vi "MainEvents.vi"() -> ()   [LabVIEW 2014]
uses:
  Commandes/Type de Mouvement PilMOT.ctl
panel:
  out "error out 2":errorcluster
  in  "Nom de base du fichier de référence Ligne à Retard":string="LigneRetard"
  in  "Nom de base du fichier de référence Miroir Troué":string="MiroirTroue"
  in  "Message":string
  in  "Nom de base du fichier de référence HeNe":string="HeNe"
  out "Axe6_Messages":u16
  out "Axe5_Messages":u16
  out "Axe4_Messages":u16
  out "Axe1_Messages":u16
  out "Axe2_Messages":u16
  out "Axe3_Messages":u16
  in  "Nom de base du fichier de références atténuateurs":string="Atténuateur"
  in  "Adresse des fichiers de référence":string="C:\\Users\\loa\\Documents\\Programmes Labview\\Moteurs Compression 5fs\\Fichiers de Référence"
  in  "STOP Moteurs":bool
  out "Adresse du PilMOT":string="ni.var.psp://localhost/OPCLib/OPC1/esbimETH_2"
  in  "stop":bool
  in  "Onglets":T1(tab)
  out "HeNe\n(µm/pas)":dbl=3.1
  out "Attenuateurs\n(µm/pas)":dbl=3.1
  out "Current LR Position \n(ps, par rapport au zéro)":dbl
  out "Butée P \n(HeNe)":bool
  out "Butée N \n(HeNe)":bool
  in  "HeNe en Butée?":bool
  in  "HeNe in?":bool
  out "PosAAtt HeNe":string
  out "HeNe":i32
  in  "HeNe Switch":bool
  out "LR (µm/pas)":dbl=3.1
  out "MT (µm/pas)":dbl=3.1
  in  "LR Deplacer":bool
  in  "LR Type Mouvement":enum16{"Absolu", "Relatif"}(ring)
  in  "LR Déplacement (µm)":dbl
  in  "MT Deplacer":bool
  in  "MT Type Mouvement":enum16{"Absolu", "Relatif"}(ring)
  in  "MT Déplacement (µm)":dbl
  in  "LR Déplacer +":bool
  in  "LR Deplacer -":bool
  in  "LR Butée +":bool
  in  "LR Butée -":bool
  in  "LR STOP mvt":bool
  in  "LR Origine ici":bool
  in  "Positions?":bool
  out "Butée P":bool[](array[boolean])
  out "Butée N":bool[](array[boolean])
  out "Position à atteindre":string[](array[string])
  in  "Actif?":bool[](array[boolean])
  in  "Att.":bool[](array[boolean])
  in  "Attenuer":bool
  out "Att. 3":i32
  out "Att. 2":i32
  out "Att. 1":i32
  in  "MT Déplacer +":bool
  in  "MT Deplacer -":bool
  in  "MT Butée +":bool
  in  "MT Butée -":bool
  in  "MT STOP mvt":bool
  in  "MT Origine ici":bool
  in  "Miroir Troué PositionCodeurEnPas":i32
  in  "Ligne à retard PositionCodeurEnPas":i32
  in  "Miroir Troué PositionTheorique":i32
  in  "Ligne à retard PositionTheorique":i32
  in  "Inversion des butées HeNe":bool=TRUE
  in  "Position HeNe":bool=TRUE
  in  "Position Laser":bool
  in  "Inversion butées":bool[](array[boolean])=[TRUE, FALSE, FALSE, FALSE]
  in  "Position Atténuateur":bool[](array[boolean])
  in  "Position Miroir":bool[](array[boolean])
  in  "Increment (mm)":dbl=0.01
  in  "Inc +":bool
  in  "Inc -":bool
  in  "Atténuateur  à référencer":T2(ring)
  in  "Set Laser":bool
  in  "Position de Référence Laser":i32
  in  "Set HeNe":bool
  in  "Position de Référence HeNe":i32
  out "Axe6_PositionTheorique":i32
  out "Axe5_PositionTheorique":i32
  out "Axe4_PositionTheorique":i32
  in  "Origine ici":bool
  in  "STOP mvt":bool
  in  "Set Atténuateur":bool
  in  "Pos. Ref. Atténuateur":i32[](array[numeric])
  in  "Set Miroir":bool
  in  "Pos. Ref. Miroir":i32[](array[numeric])
  in  "Moteur à déplacer":T3(ring)
  in  "Butée -":bool
  in  "Butée +":bool
  in  "Deplacer -":bool
  in  "Déplacer +":bool
  out "Axe3_PositionTheorique":i32
  out "Axe2_PositionTheorique":i32
  out "Axe1_PositionTheorique":i32
  out "Axe6_PositionTheorique 2":i32
  out "Axe5_PositionTheorique 2":i32
  in  "Go to ref":bool
  in  "Set ref":bool
  in  "Numéro de Pos. Ref.":T4(ring)
  in  "Ref. Tab. Origine ici":bool
  in  "Ref. Tab STOP mvt":bool
  in  "Ref. Tab Butée -":bool
  in  "Ref. Tab Butée +":bool
  in  "Ref. Tab Deplacer -":bool
  in  "Ref. Tab Déplacer +":bool
  in  "Moteur à référencer":T5(ring)
  in  "Libellés pos. de référence":string[](array[string])
  out "Positions de référence":i32[](array[numeric])
  out "Axe1_PositionTheorique 2":i32
  out "Axe2_PositionTheorique 2":i32
  out "Axe3_PositionTheorique 2":i32
  out "Axe4_PositionTheorique 2":i32
  out "error out":errorcluster
  in  "error in":errorcluster
  # "Should be working now... :D"
  # "Message Axes"
  # "Attenuation"
  # "Positions à atteindre"
  # "Positions actuelles"
  # "Att1 (M1)"
  # "Att2 (M2)"
  # "Att3 (M3)"
  # "HeNe (M4)"
  # "Position à atteindre"
  # "Position actuelle"
  # "Miroir Troué (M5)"
  # "Near Field Mirror (M6)"
  # "Position butée/position de référence atténuateurs"
  # "Position Miroir\n(butée/pos.ref.)"
  # "Position Atténuateur\n(butée/pos.ref.)"
  # "Inversion des butées\n(Normal/Inversé)"
  # "Position butée/position de référence HeNe"
  # "Positions moteurs \n(théorique, en pas)"
  # "Att. 1"
  # "Att. 2"
  # "Procédure de référencement des moteurs:"
  # "Att. 3"
  # "HeNe"
  # "Miroir Troué"
  # "1. Aller en butée -\n2. Faire le zéro\n3. Déplacer jusqu'en pos. ref\n4. Set"
  # "Delay Line"
  # "Pos. ref. Miroir\n(théorique, en pas)"
  # "Pos. ref. Atténuateur\n(théorique, en pas)"
  # "Att. 1"
  # "Att. 2"
  # "Att. 3"
  # "Pos. ref. HeNe\n(théorique, en pas)"
  # "Pos. ref. Laser\n(théorique, en pas)"
  # "HeNe"
  # "Références tous moteurs"
  # "Position actuelle"
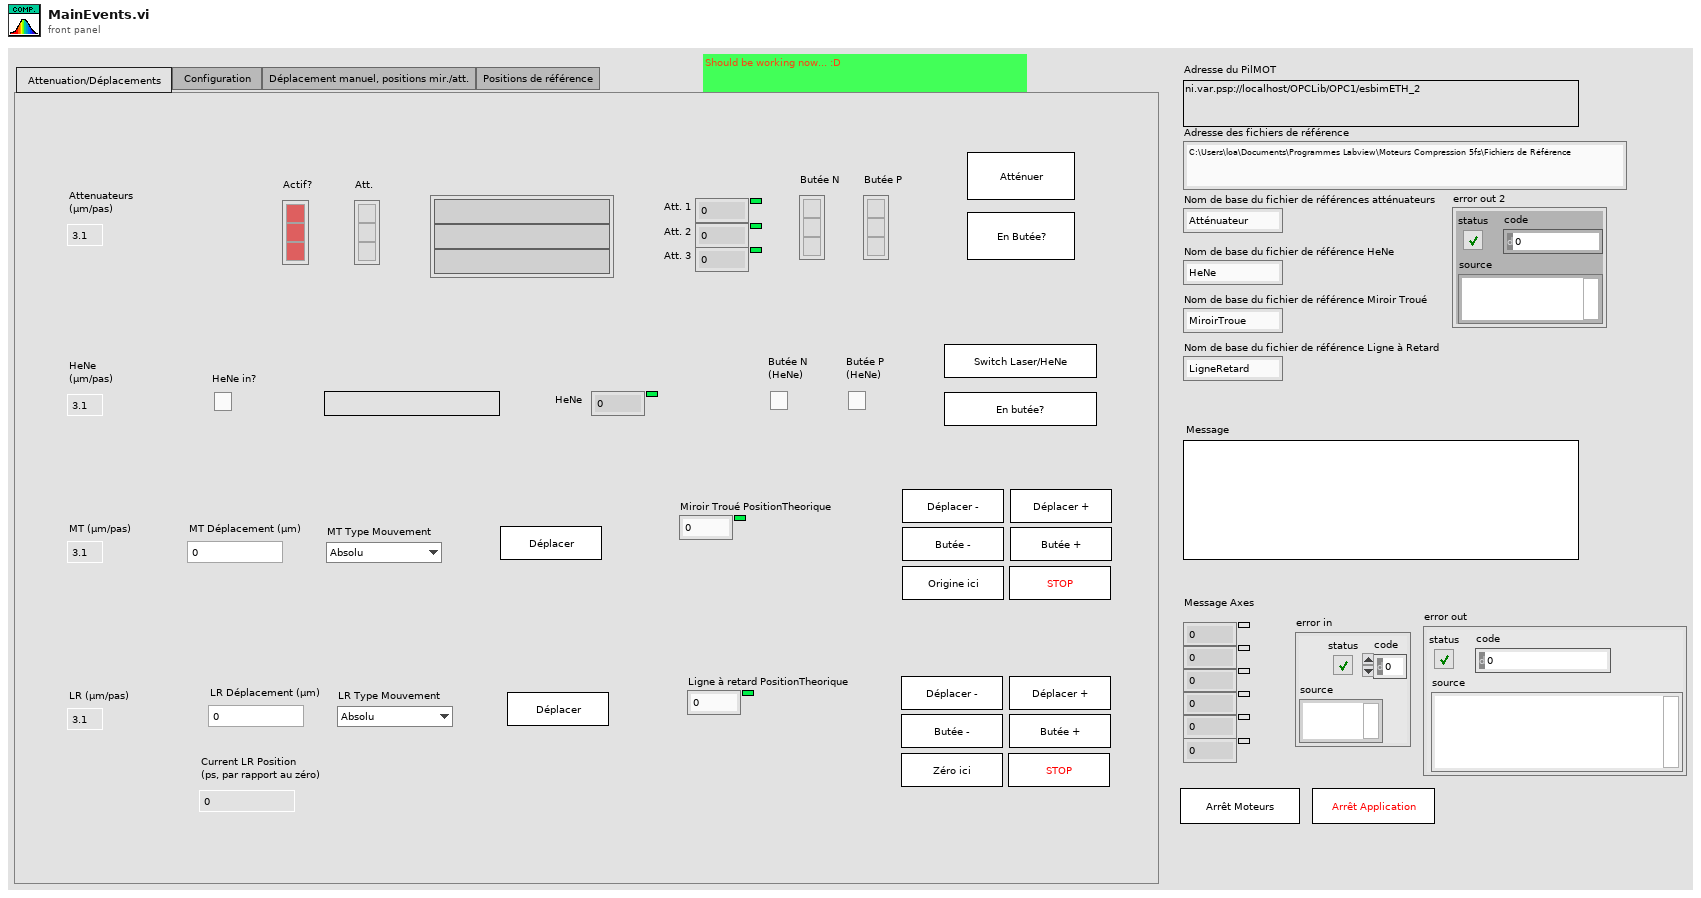
[diagram p1: front panel]
types:
  T1 = enum32{"Attenuation/Déplacements   ", "Configuration   ", "Déplacement manuel, positions mir./att.", "Positions de référence"}
  T2 = enum16{"Atténuateur 1", "Atténuateur 2", "Atténuateur 3"}
  T3 = enum16{"Atténuateur 1", "Atténuateur 2", "Atténuateur 3", "HeNe", "Miroir Troué", "Delay Line"}
  T4 = enum16{"Position 1", "Position 2", "Position 3", "Position 4"}
  T5 = enum16{"Atténuateur 1", "Atténuateur 2", "Atténuateur 3", "HeNe", "Miroir Troué", "Ligne à Retard"}
  T6 = enum16{"open", "replace", "create", "open or create", "replace or create", "replace or create with confirmation"}
  T7 = typedef "Type de Mouvement PilMOT.ctl" = u16
  T8 = typedef "AdressesVariablesPartagees.ctl" = cluster{"OrdreBloc":string, "Ordre UC":string, "CoteAAtteindre":string, "Vitesse":string, "Position codeur en pas":string, "Position Théorique":string, "Message":string, "Ecrire":string, "Zone à écrire":string, "Numéro paramètre":string, "Ordre":string, "Valeur":string, "Valeur Lecture":string, "Numéro paramètre Lecture":string, "Acquittement Lecture Ecriture":string, "Zone à Ecrire Pour Axe ":u16, "Acquittement Ordre UC":string}
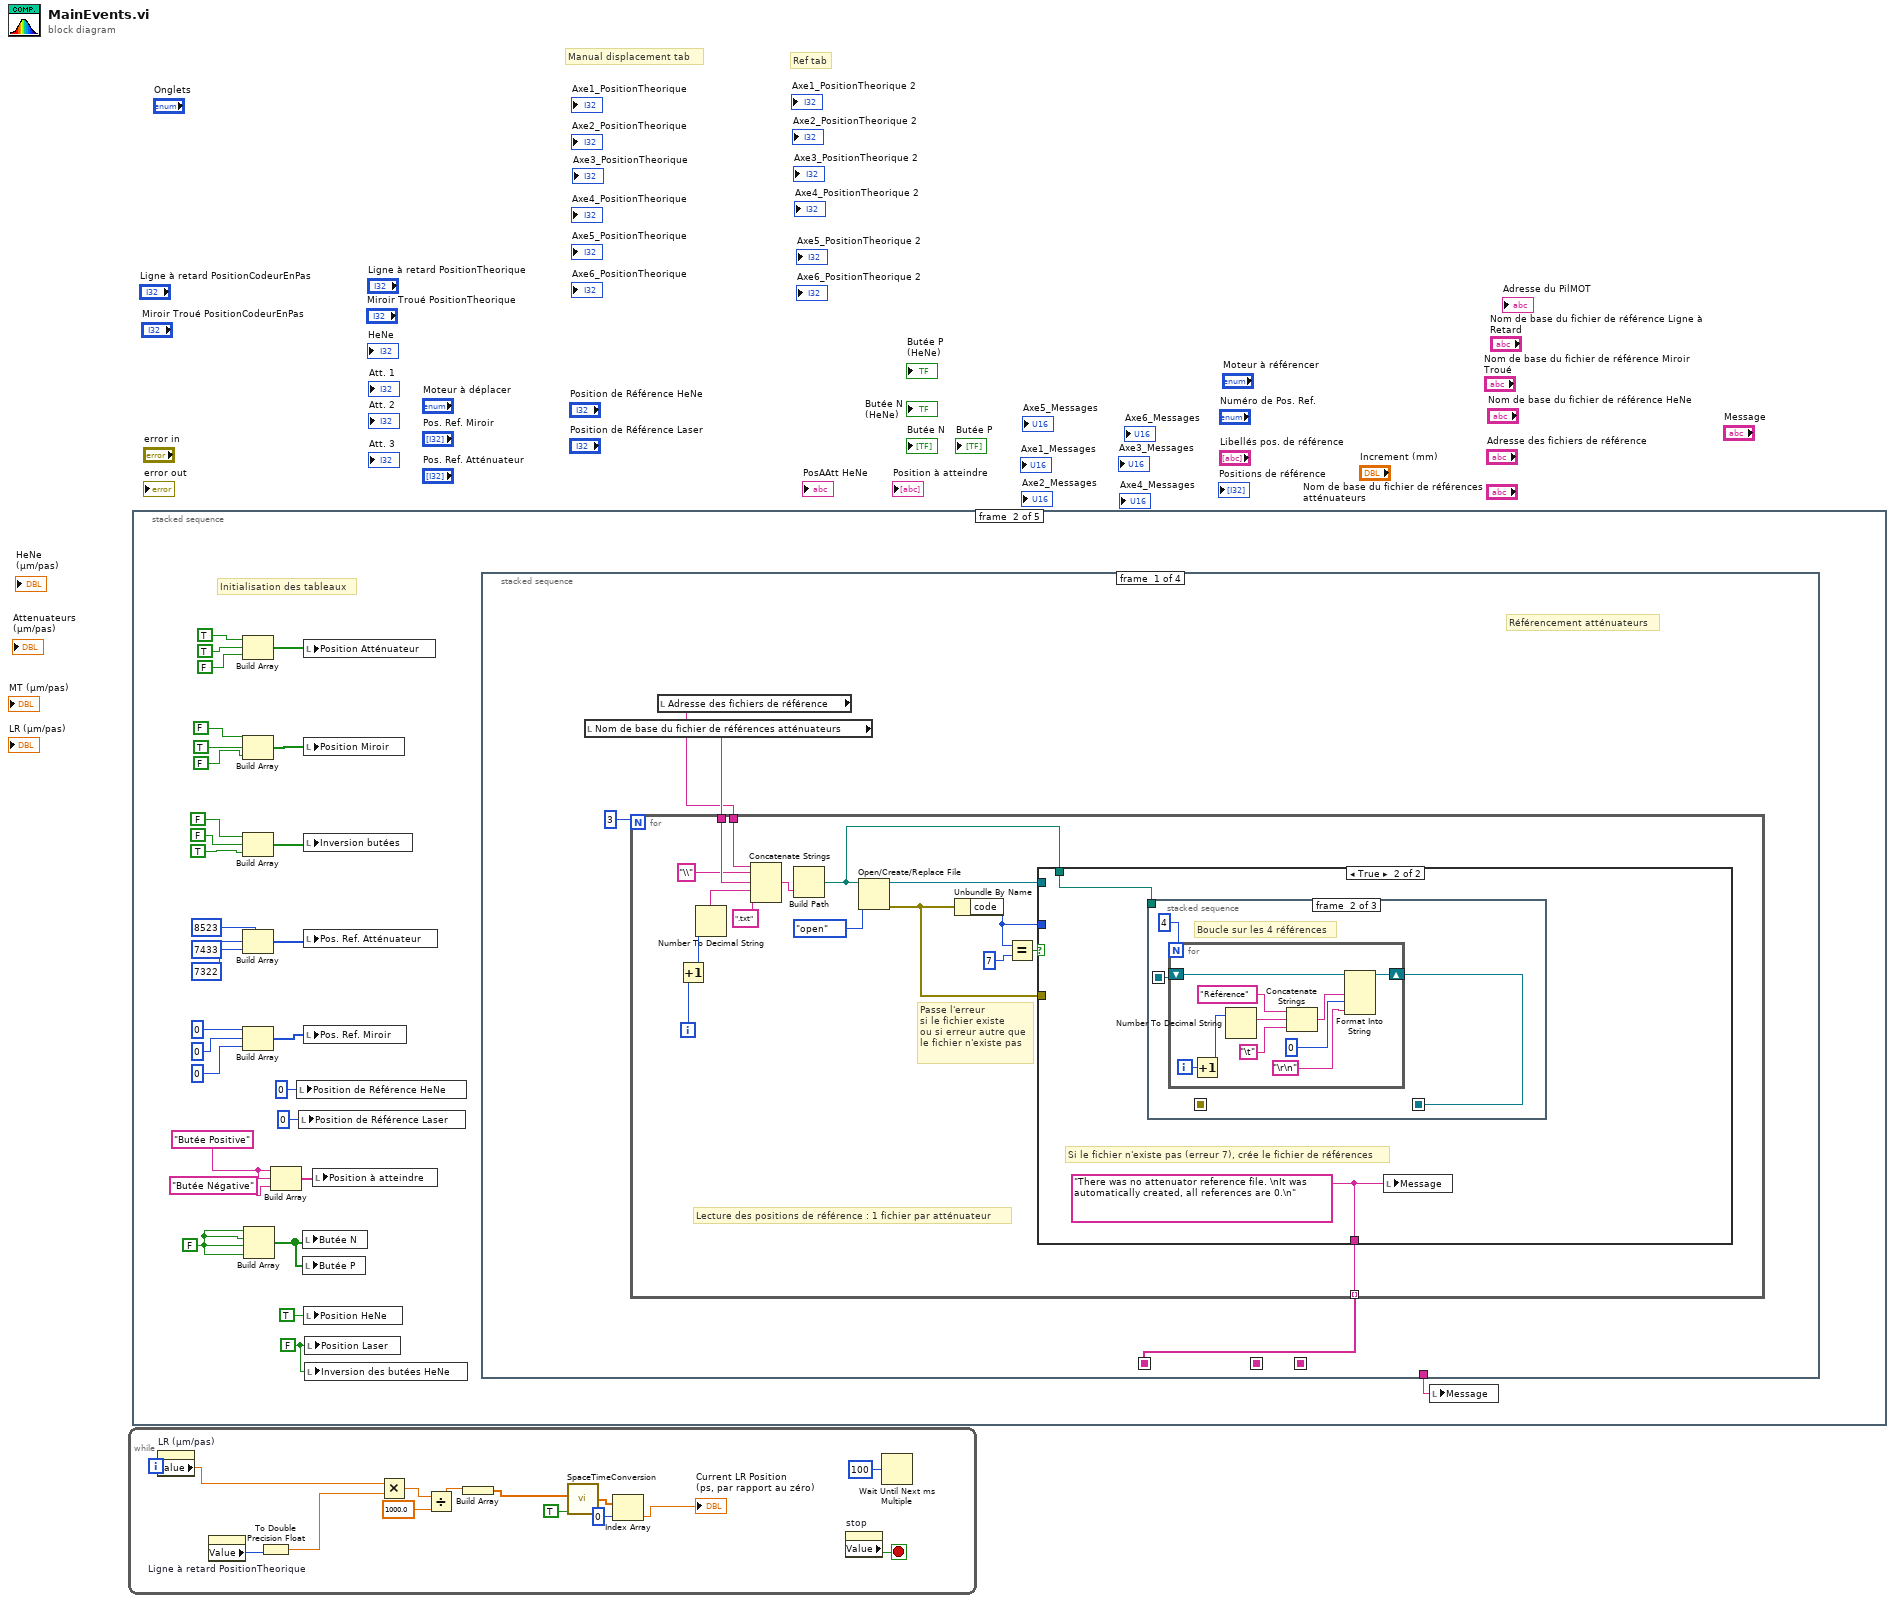
[diagram p0: block diagram]
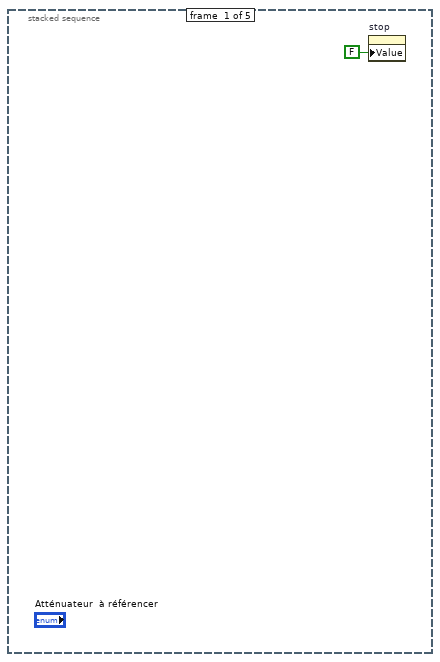
[diagram p2: hidden frame]
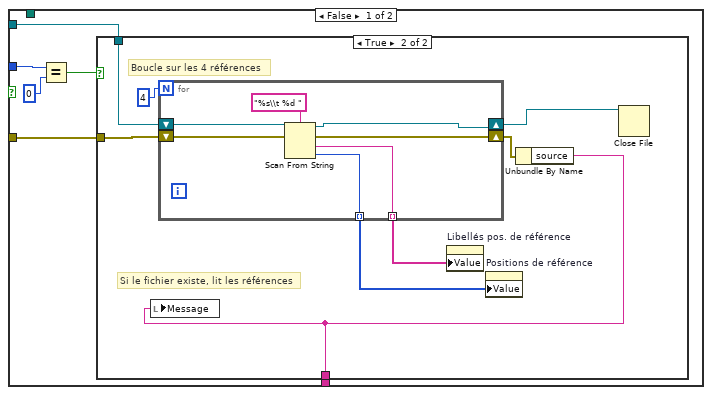
[diagram p3: hidden frame]
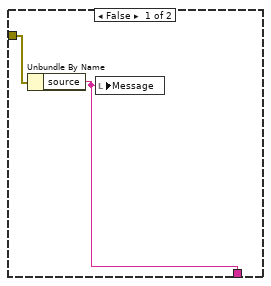
[diagram p4: hidden frame]
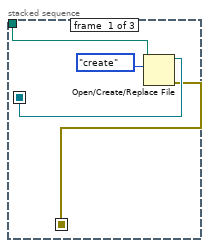
[diagram p5: hidden frame]
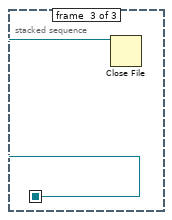
[diagram p6: hidden frame]
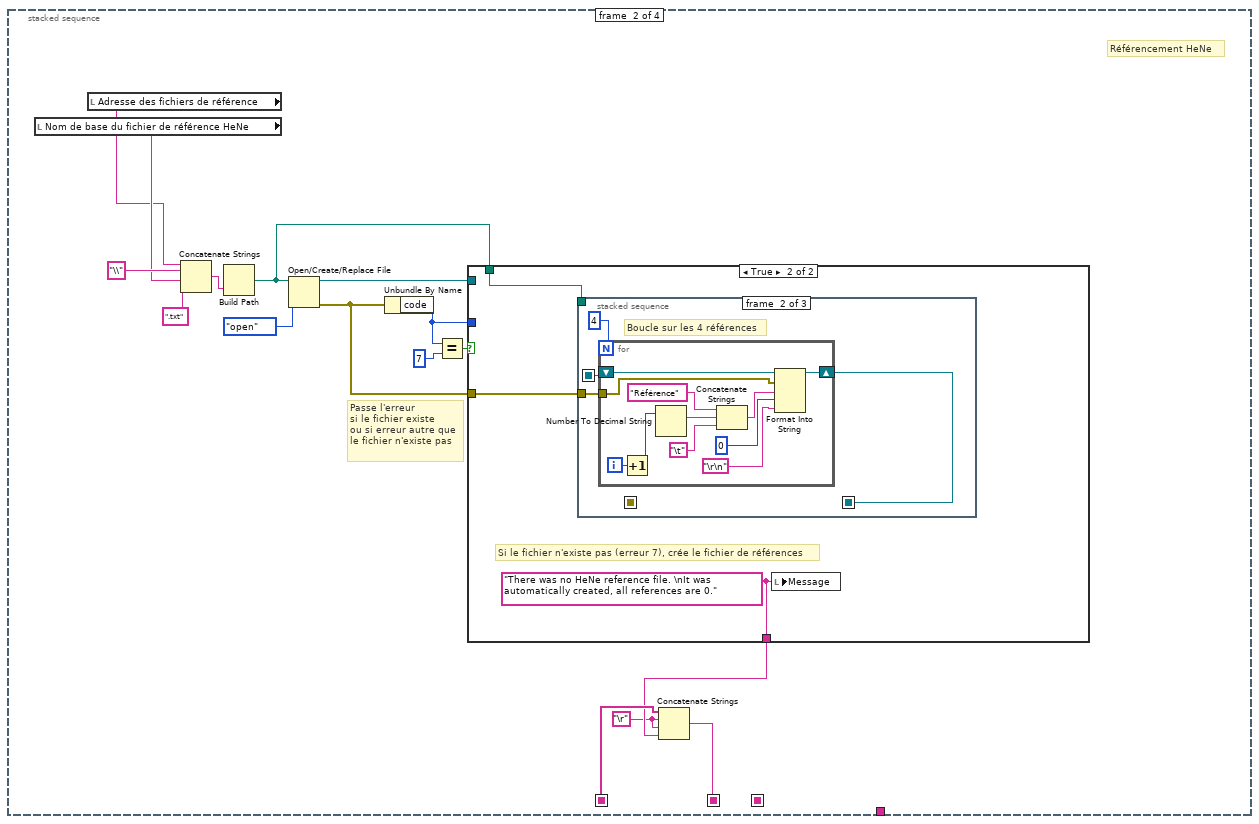
[diagram p7: hidden frame]
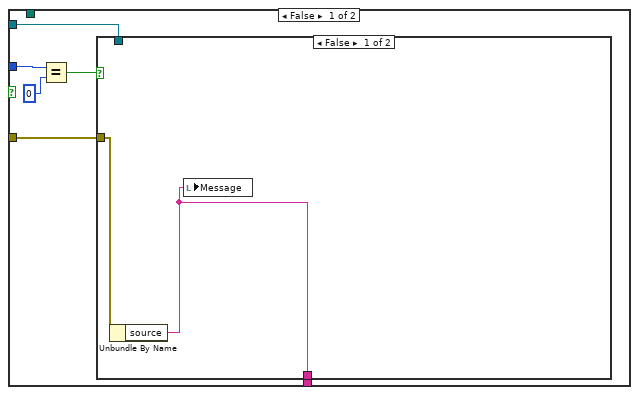
[diagram p8: hidden frame]
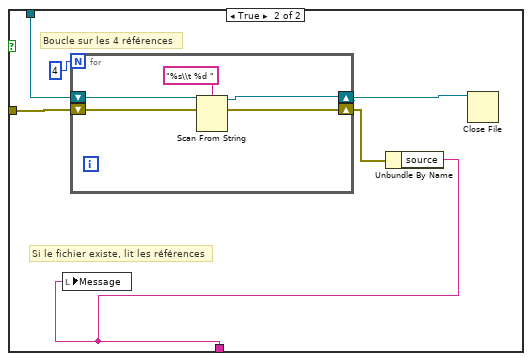
[diagram p9: hidden frame]
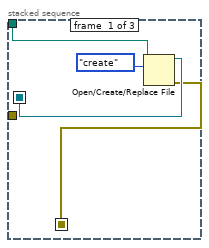
[diagram p10: hidden frame]
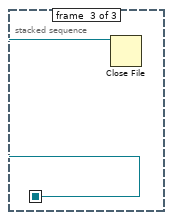
[diagram p11: hidden frame]
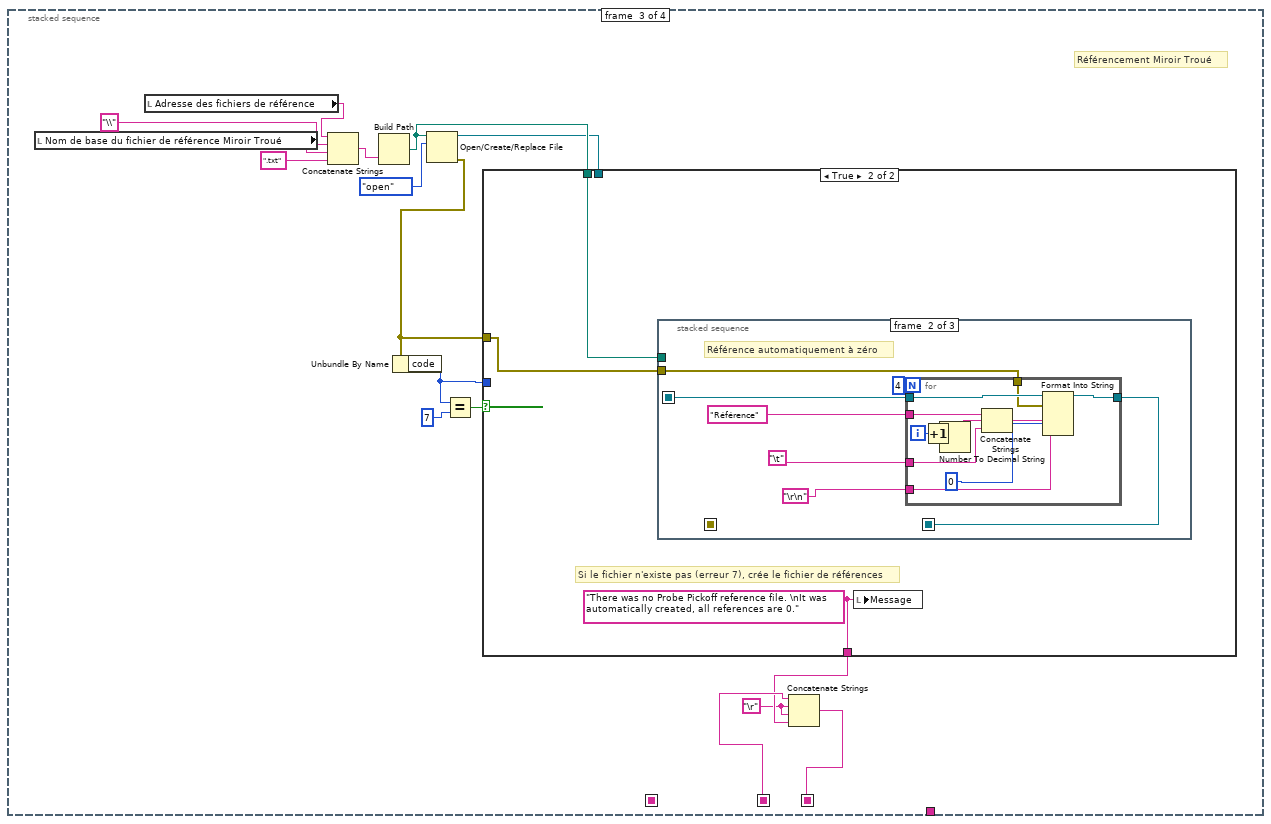
[diagram p12: hidden frame]
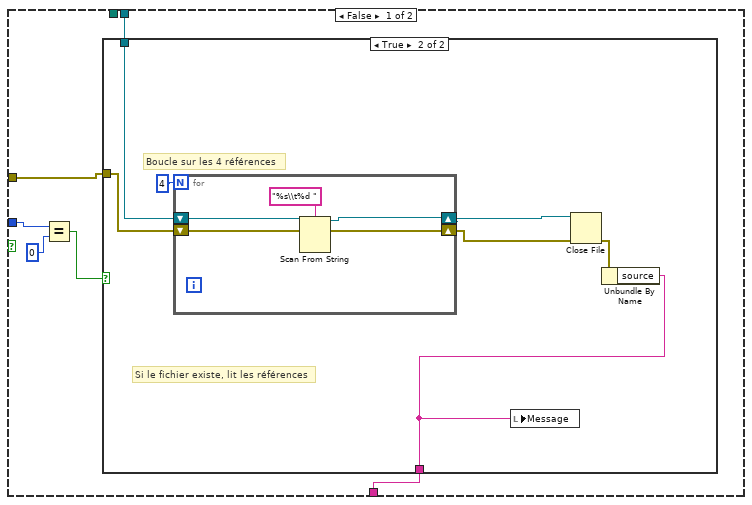
[diagram p13: hidden frame]
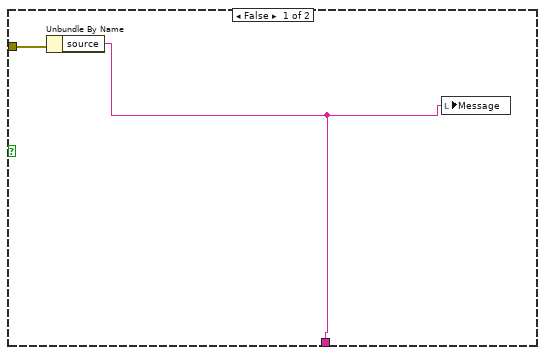
[diagram p14: hidden frame]
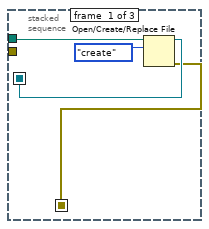
[diagram p15: hidden frame]
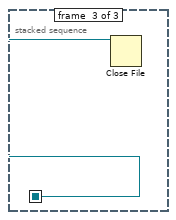
[diagram p16: hidden frame]
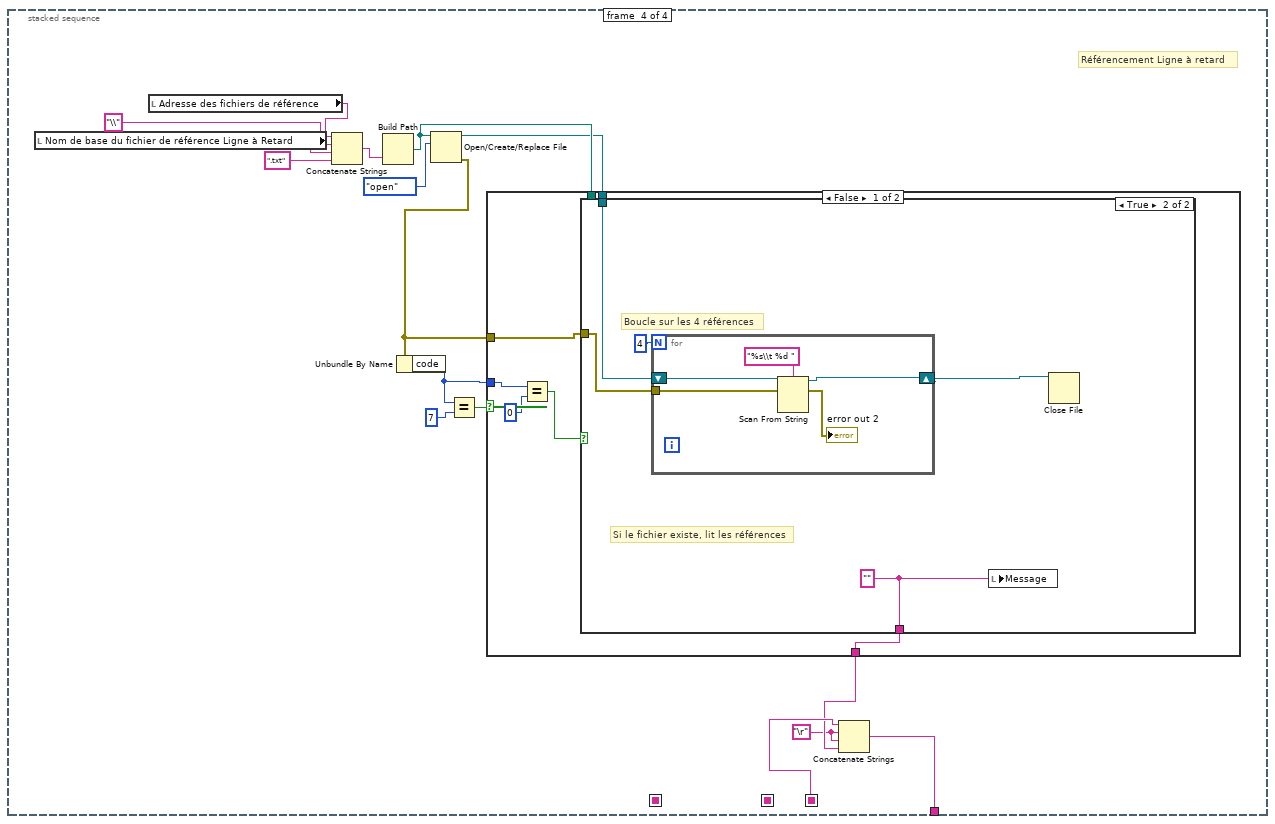
[diagram p17: hidden frame]
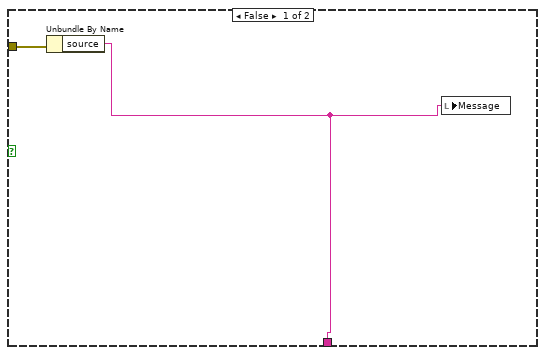
[diagram p18: hidden frame]
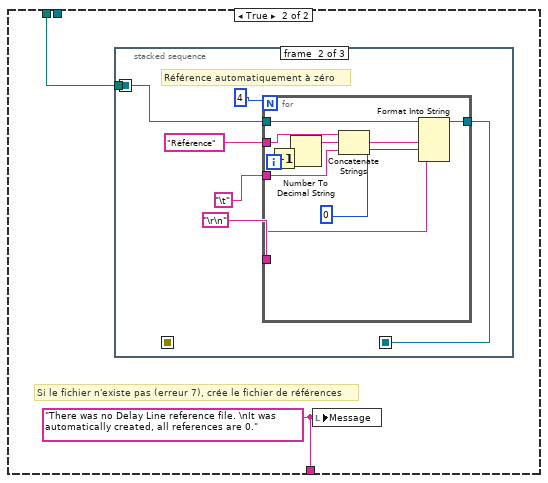
[diagram p19: hidden frame]
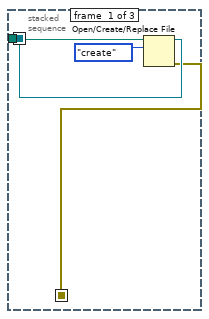
[diagram p20: hidden frame]
diagram:
  # "Ref tab"
  # "Manual displacement tab"
  n1 = while {
    stop <- w13 stop-if-true
    n2 = property on="LR (µm/pas)" class="DigNum (strict)"() -> ("Value"=w11:dbl)  [unwired: 2 in, 2 out]
    n3 = property on="Ligne à retard PositionTheorique" class="DigNum (strict)"() -> ("Value"=w10:i32)  [unwired: 2 in, 2 out]
    n4 = To Double Precision Float(number=w10) -> (double precision float=w9:dbl)
    n5 = Multiply(x=w11, y=w9) -> (x*y=w4:dbl)
    n6 = Divide(x=w4, y=1000.0) -> (x/y=w2:dbl)
    n7 = Build Array(w2) -> (w3:dbl[])
    n8 = call "SpaceTimeConversion.vi"("Conversion Type: T : Distance to Time\n                             F : Time to Distance"=TRUE ("Conversion Type: T : Distance to Time\n                             F : Time to Distance"), "Distance IN (mm)"=w3) -> ("Time OUT (ps) / Distance OUT (mm)"=w7:dbl[])  [unwired: 2 in]
    n9 = Index Array(array=w7, index=0) -> (element=→"Current LR Position \n(ps, par rapport au zéro)":dbl)
    n10 = property on="stop" class="Bool (strict)"() -> ("Value"=w13:bool)  [unwired: 2 in, 2 out]
    n11 = Wait Until Next ms Multiple(millisecond multiple=u32 100) -> ()  [unwired: 1 out]
  }
  n12 = stacked-sequence {
    frame #0 {
      n13 = property on="stop" class="Bool (strict)"("Value"=FALSE ("stop")) -> ()  [unwired: 2 in, 2 out]
    }
    frame #1 {
      w18 = FALSE ("Position Laser")
      w20 = "Butée Positive"
      w23 = FALSE
      # "Initialisation des tableaux"
      n14 = Build Array(TRUE, TRUE, FALSE) -> (w41:bool[])
      n15 = Build Array(FALSE, TRUE, FALSE) -> (w37:bool[])
      n16 = Build Array(FALSE, FALSE, TRUE) -> (w33:bool[])
      n17 = Build Array(8523, 7433, 7322) -> (w25:i32[])
      n18 = Build Array(0, 0, 0) -> (w32:i32[])
      n19 = Build Array(w23, w23, w23, w23) -> (w22:bool[])
      n20 = Build Array(w20, w20, "Butée Négative") -> (w24:string[])
      n21 = local write "Position de Référence HeNe"(0 ("Position de Référence HeNe")) -> ()
      n22 = local write "Position de Référence Laser"(0 ("Position de Référence Laser")) -> ()
      n23 = local write "Butée N"(w22) -> ()
      n24 = local write "Butée P"(w22) -> ()
      n25 = local write "Position Atténuateur"(w41) -> ()
      n26 = local write "Position Miroir"(w37) -> ()
      n27 = local write "Inversion butées"(w33) -> ()
      n28 = local write "Pos. Ref. Atténuateur"(w25) -> ()
      n29 = local write "Pos. Ref. Miroir"(w32) -> ()
      n30 = local write "Position HeNe"(TRUE ("Position HeNe")) -> ()
      n31 = local write "Position Laser"(w18) -> ()
      n32 = local write "Inversion des butées HeNe"(w18) -> ()
      n33 = local write "Position à atteindre"(w24) -> ()
      n34 = stacked-sequence {
        seq-local: [w45 _ _ _] -> [_ w111 _ _]
        seq-local: [_ w109 _ _] -> [_ _ w169 _]
        seq-local: [_ _ w167 _] -> [_ _ _ w231]
        tunnel: [_ _ _ w229] -> w15
        frame #0 {
          # "Référencement atténuateurs"
          n35 = local read "Nom de base du fichier de références atténuateurs"() -> (w47:string)
          n36 = local read "Adresse des fichiers de référence"() -> (w46:string)
          n37 = for {
            N: 3 -> [_]
            tunnel: w46 -> [w52]
            tunnel: w47 -> [w53]
            tunnel: [w49] -> w45 mode=indexing
            i -> [w64]
            # "Lecture des positions de référence : 1 fichier par atténuateur"
            # "Passe l'erreur\nsi le fichier existe\nou si erreur autre que\nle fichier n'existe pas"
            n38 = Increment(x=w64) -> (x+1=w50:i32)
            n39 = Number To Decimal String(number=w50) -> (decimal integer string=w63:string)  [unwired: 1 in]
            n40 = Concatenate Strings(w52, "\\", w53, w63, ".txt" ("string")) -> (w61:string)
            n41 = Build Path(name or relative path=w61) -> (appended path=w57:path)  [unwired: 1 in]
            n42 = Open/Create/Replace File(file path (use dialog)=w57, operation (0:open)=T6."open") -> (refnum out=w55:refnum<file>, error out=w54:errorcluster)  [unwired: 4 in, 1 out]
            n43 = Unbundle By Name(w54) -> ("code"=w56:i32)
            n44 = Equal?(x=w56, y=7) -> (x = y?=w58:bool)
            n45 = case shown="True" w58 {
              tunnel: w57 -> [_ w89]
              tunnel: w56 -> [w70 _]
              tunnel: w55 -> [w67 _]
              tunnel: w54 -> [w66 _]
              tunnel: [w65 w88] -> w49
              frame False {
                n46 = Equal?(x=w70, y=0) -> (x = y?=w68:bool)
                n47 = case shown="True" w68 {
                  tunnel: w67 -> [_ w79]
                  tunnel: w66 -> [w72 w78]
                  tunnel: [w71 w73] -> w65
                  frame False {
                    n48 = Unbundle By Name(w72) -> ("source"=w71:string)
                    n49 = local write "Message"(w71) -> ()
                  }
                  frame True {
                    # "Si le fichier existe, lit les références"
                    # "Boucle sur les 4 références"
                    n50 = for {
                      N: 4 -> [_]
                      shift-right: [w85] -> w77
                      shift-left: w79 -> [w87]
                      tunnel: [w83] -> w76 mode=indexing
                      tunnel: [w82] -> w75 mode=indexing
                      shift-right: [w81] -> w74
                      shift-left: w78 -> [w86]
                      n51 = Scan From String("%s\\t %d " ("format string"), w87, w86) -> (w85:refnum<file>, w81:errorcluster, output 1=w83:string, output 2=w82:i32)  [unwired: 2 in]
                    }
                    n52 = property on="Libellés pos. de référence" class="Arr (strict)"("Value"=w76) -> ()  [unwired: 2 in, 2 out]
                    n53 = property on="Positions de référence" class="Arr (strict)"("Value"=w75) -> ()  [unwired: 2 in, 2 out]
                    n54 = Unbundle By Name(w74) -> ("source"=w73:string)
                    n55 = local write "Message"(w73) -> ()
                    n56 = Close File(refnum=w77) -> ()  [unwired: 1 in, 2 out]
                  }
                }
              }
              frame True {
                w88 = "There was no attenuator reference file. \nIt was automatically created, all references are 0.\n" ("Message")
                # "Si le fichier n'existe pas (erreur 7), crée le fichier de références"
                n57 = stacked-sequence {
                  seq-local: [w91 _ _] -> [_ w94 _]
                  seq-local: [w90 _ _] -> [_ _ _]
                  seq-local: [_ w95 _] -> [_ _ w107]
                  tunnel: w89 -> [w93 _ _]
                  frame #0 {
                    n58 = Open/Create/Replace File(file path (use dialog)=w93, operation (0:open)=T6."create") -> (refnum out=w91:refnum<file>, error out=w90:errorcluster)  [unwired: 4 in, 1 out]
                  }
                  frame #1 {
                    # "Boucle sur les 4 références"
                    n59 = for {
                      N: 4 -> [_]
                      shift-right: [w105] -> w95
                      shift-left: w94 -> [w106]
                      i -> [w104]
                      n60 = Increment(x=w104) -> (x+1=w97:i32)
                      n61 = Number To Decimal String(number=w97) -> (decimal integer string=w103:string)  [unwired: 1 in]
                      n62 = Concatenate Strings("Référence", w103, "\t") -> (w101:string)
                      n63 = Format Into String(initial string=w106, w101, 0, "\r\n") -> (resulting string=w105:refnum<file>)  [unwired: 2 in, 1 out]
                    }
                  }
                  frame #2 {
                    n64 = Close File(refnum=w107) -> ()  [unwired: 1 in, 2 out]
                  }
                }
                n65 = local write "Message"(w88) -> ()
              }
            }
          }
        }
        frame #1 {
          w108 = "\r"
          # "Passe l'erreur\nsi le fichier existe\nou si erreur autre que\nle fichier n'existe pas"
          # "Référencement HeNe"
          n66 = local read "Nom de base du fichier de référence HeNe"() -> (w113:string)
          n67 = local read "Adresse des fichiers de référence"() -> (w112:string)
          n68 = Concatenate Strings(w112, "\\", w113, ".txt" ("string")) -> (w115:string)
          n69 = Build Path(name or relative path=w115) -> (appended path=w119:path)  [unwired: 1 in]
          n70 = Open/Create/Replace File(file path (use dialog)=w119, operation (0:open)=T6."open") -> (refnum out=w121:refnum<file>, error out=w122:errorcluster)  [unwired: 4 in, 1 out]
          n71 = Unbundle By Name(w122) -> ("code"=w120:i32)
          n72 = Equal?(x=w120, y=7) -> (x = y?=w118:bool)
          n73 = case shown="True" w118 {
            tunnel: w119 -> [_ w145]
            tunnel: w120 -> [w129 _]
            tunnel: w121 -> [w126 _]
            tunnel: w122 -> [w125 w143]
            tunnel: [w124 w144] -> w110
            frame False {
              n74 = Equal?(x=w129, y=0) -> (x = y?=w127:bool)
              n75 = case shown="False" w127 {
                tunnel: w126 -> [_ w136]
                tunnel: w125 -> [w131 w135]
                tunnel: [w130 w132] -> w124
                frame False {
                  n76 = Unbundle By Name(w131) -> ("source"=w130:string)
                  n77 = local write "Message"(w130) -> ()
                }
                frame True {
                  # "Si le fichier existe, lit les références"
                  # "Boucle sur les 4 références"
                  n78 = for {
                    N: 4 -> [_]
                    shift-right: [w140] -> w134
                    shift-left: w136 -> [w142]
                    shift-right: [w138] -> w133
                    shift-left: w135 -> [w141]
                    n79 = Scan From String("%s\\t %d " ("format string"), w142, w141) -> (w140:refnum<file>, w138:errorcluster)  [unwired: 4 in]
                  }
                  n80 = Unbundle By Name(w133) -> ("source"=w132:string)
                  n81 = local write "Message"(w132) -> ()
                  n82 = Close File(refnum=w134) -> ()  [unwired: 1 in, 2 out]
                }
              }
            }
            frame True {
              w144 = "There was no HeNe reference file. \nIt was automatically created, all references are 0." ("Message")
              # "Si le fichier n'existe pas (erreur 7), crée le fichier de références"
              n83 = stacked-sequence {
                seq-local: [w147 _ _] -> [_ w151 _]
                seq-local: [w146 _ _] -> [_ _ _]
                seq-local: [_ w152 _] -> [_ _ w165]
                tunnel: w145 -> [w149 _ _]
                tunnel: w143 -> [_ w150 _]
                frame #0 {
                  n84 = Open/Create/Replace File(file path (use dialog)=w149, operation (0:open)=T6."create") -> (refnum out=w147:refnum<file>, error out=w146:errorcluster)  [unwired: 4 in, 1 out]
                }
                frame #1 {
                  # "Boucle sur les 4 références"
                  n85 = for {
                    N: 4 -> [_]
                    shift-right: [w163] -> w152
                    shift-left: w151 -> [w164]
                    tunnel: w150 -> [w154]
                    i -> [w162]
                    n86 = Increment(x=w162) -> (x+1=w155:i32)
                    n87 = Number To Decimal String(number=w155) -> (decimal integer string=w161:string)  [unwired: 1 in]
                    n88 = Concatenate Strings("Référence", w161, "\t") -> (w159:string)
                    n89 = Format Into String(initial string=w164, error in=w154, w159, 0, "\r\n") -> (resulting string=w163:refnum<file>)  [unwired: 1 in, 1 out]
                  }
                }
                frame #2 {
                  n90 = Close File(refnum=w165) -> ()  [unwired: 1 in, 2 out]
                }
              }
              n91 = local write "Message"(w144) -> ()
            }
          }
          n92 = Concatenate Strings(w111, w108, w108, w110) -> (w109:string)
        }
        frame #2 {
          w166 = "\r"
          # "Référencement Miroir Troué"
          n93 = local read "Nom de base du fichier de référence Miroir Troué"() -> (w179:string)
          n94 = local read "Adresse des fichiers de référence"() -> (w181:string)
          n95 = Concatenate Strings(w181, "\\", w179, ".txt" ("string")) -> (w177:string)
          n96 = Build Path(name or relative path=w177) -> (appended path=w173:path)  [unwired: 1 in]
          n97 = Open/Create/Replace File(file path (use dialog)=w173, operation (0:open)=T6."open") -> (refnum out=w171:refnum<file>, error out=w170:errorcluster)  [unwired: 4 in, 1 out]
          n98 = Unbundle By Name(w170) -> ("code"=w172:i32)
          n99 = Equal?(x=w172, y=7) -> (x = y?=w174:bool)
          n100 = case shown="True" w174 {
            tunnel: w173 -> [_ w204]
            tunnel: w172 -> [w186 _]
            tunnel: w171 -> [w184 _]
            tunnel: w170 -> [w183 w202]
            tunnel: [w182 w203] -> w168
            frame False {
              n101 = Equal?(x=w186, y=0) -> (x = y?=w185:bool)
              n102 = case shown="True" w185 {
                tunnel: w184 -> [_ w195]
                tunnel: w183 -> [w189 w193]
                tunnel: [w188 w190] -> w182
                frame False {
                  n103 = Unbundle By Name(w189) -> ("source"=w188:string)
                  n104 = local write "Message"(w188) -> ()
                }
                frame True {
                  # "Si le fichier existe, lit les références"
                  # "Boucle sur les 4 références"
                  n105 = for {
                    N: 4 -> [_]
                    shift-right: [w200] -> w194
                    shift-left: w195 -> [w201]
                    shift-right: [w197] -> w192
                    shift-left: w193 -> [w198]
                    n106 = Scan From String("%s\\t%d " ("format string"), w201, w198) -> (w200:refnum<file>, w197:errorcluster)  [unwired: 4 in]
                  }
                  n107 = Close File(refnum=w194, error in=w192) -> (error out=w191:errorcluster)  [unwired: 1 out]
                  n108 = Unbundle By Name(w191) -> ("source"=w190:string)
                  n109 = local write "Message"(w190) -> ()
                }
              }
            }
            frame True {
              w203 = "There was no Probe Pickoff reference file. \nIt was automatically created, all references are 0." ("Message")
              # "Si le fichier n'existe pas (erreur 7), crée le fichier de références"
              n110 = stacked-sequence {
                seq-local: [w207 _ _] -> [_ w214 _]
                seq-local: [w206 _ _] -> [_ _ _]
                seq-local: [_ w215 _] -> [_ _ w227]
                tunnel: w204 -> [w205 _ _]
                tunnel: w202 -> [_ w209 _]
                frame #0 {
                  n111 = Open/Create/Replace File(file path (use dialog)=w205, operation (0:open)=T6."create") -> (refnum out=w207:refnum<file>, error out=w206:errorcluster)  [unwired: 4 in, 1 out]
                }
                frame #1 {
                  # "Référence automatiquement à zéro"
                  n112 = for {
                    N: 4 -> [_]
                    tunnel: [w226] -> w215
                    tunnel: w214 -> [w225]
                    tunnel: "\r\n" -> [w222]
                    tunnel: "Référence" -> [w219]
                    tunnel: "\t" -> [w217]
                    tunnel: w209 -> [w216]
                    i -> [w224]
                    n113 = Increment(x=w224) -> (x+1=w221:i32)
                    n114 = Number To Decimal String(number=w221) -> (decimal integer string=w220:string)  [unwired: 1 in]
                    n115 = Concatenate Strings(w219, w220, w217) -> (w218:string)
                    n116 = Format Into String(initial string=w225, error in=w216, w218, 0, w222) -> (resulting string=w226:refnum<file>)  [unwired: 1 in, 1 out]
                  }
                }
                frame #2 {
                  n117 = Close File(refnum=w227) -> ()  [unwired: 1 in, 2 out]
                }
              }
              n118 = local write "Message"(w203) -> ()
            }
          }
          n119 = Concatenate Strings(w169, w166, w166, w168) -> (w167:string)
        }
        frame #3 {
          w228 = "\r"
          # "Référencement Ligne à retard"
          n120 = local read "Nom de base du fichier de référence Ligne à Retard"() -> (w241:string)
          n121 = local read "Adresse des fichiers de référence"() -> (w243:string)
          n122 = Concatenate Strings(w243, "\\", w241, ".txt" ("string")) -> (w239:string)
          n123 = Build Path(name or relative path=w239) -> (appended path=w235:path)  [unwired: 1 in]
          n124 = Open/Create/Replace File(file path (use dialog)=w235, operation (0:open)=T6."open") -> (refnum out=w233:refnum<file>, error out=w232:errorcluster)  [unwired: 4 in, 1 out]
          n125 = Unbundle By Name(w232) -> ("code"=w234:i32)
          n126 = Equal?(x=w234, y=7) -> (x = y?=w236:bool)
          n127 = case shown="False" w236 {
            tunnel: w235 -> [_ w263]
            tunnel: w234 -> [w248 _]
            tunnel: w233 -> [w246 _]
            tunnel: w232 -> [w245 _]
            tunnel: [w244 w262] -> w230
            frame False {
              n128 = Equal?(x=w248, y=0) -> (x = y?=w247:bool)
              n129 = case shown="True" w247 {
                tunnel: w246 -> [_ w255]
                tunnel: w245 -> [w251 w252]
                tunnel: [w250 w253] -> w244
                frame False {
                  n130 = Unbundle By Name(w251) -> ("source"=w250:string)
                  n131 = local write "Message"(w250) -> ()
                }
                frame True {
                  w253 = "" ("Message")
                  # "Si le fichier existe, lit les références"
                  # "Boucle sur les 4 références"
                  n132 = for {
                    N: 4 -> [_]
                    shift-right: [w260] -> w254
                    shift-left: w255 -> [w261]
                    tunnel: w252 -> [w258]
                    n133 = Scan From String("%s\\t %d " ("format string"), w261, w258) -> (w260:refnum<file>, →"error out 2":errorcluster)  [unwired: 4 in]
                  }
                  n134 = local write "Message"(w253) -> ()
                  n135 = Close File(refnum=w254) -> ()  [unwired: 1 in, 2 out]
                }
              }
            }
            frame True {
              w262 = "There was no Delay Line reference file. \nIt was automatically created, all references are 0." ("Message")
              # "Si le fichier n'existe pas (erreur 7), crée le fichier de références"
              n136 = stacked-sequence {
                seq-local: [w266 _ _] -> [_ w272 _]
                seq-local: [w265 _ _] -> [_ _ _]
                seq-local: [_ w273 _] -> [_ _ w284]
                tunnel: w263 -> [w264 _ _]
                frame #0 {
                  n137 = Open/Create/Replace File(file path (use dialog)=w264, operation (0:open)=T6."create") -> (refnum out=w266:refnum<file>, error out=w265:errorcluster)  [unwired: 4 in, 1 out]
                }
                frame #1 {
                  # "Référence automatiquement à zéro"
                  n138 = for {
                    N: 4 -> [_]
                    tunnel: [w283] -> w273
                    tunnel: w272 -> [w282]
                    tunnel: "\r\n" -> [w279]
                    tunnel: "Référence" -> [w276]
                    tunnel: "\t" -> [w274]
                    i -> [w281]
                    n139 = Increment(x=w281) -> (x+1=w278:i32)
                    n140 = Number To Decimal String(number=w278) -> (decimal integer string=w277:string)  [unwired: 1 in]
                    n141 = Concatenate Strings(w276, w277, w274) -> (w275:string)
                    n142 = Format Into String(initial string=w282, w275, 0, w279) -> (resulting string=w283:refnum<file>)  [unwired: 2 in, 1 out]
                  }
                }
                frame #2 {
                  n143 = Close File(refnum=w284) -> ()  [unwired: 1 in, 2 out]
                }
              }
              n144 = local write "Message"(w262) -> ()
            }
          }
          n145 = Concatenate Strings(w231, w228, w228, w230) -> (w229:string)
        }
      }
      n146 = local write "Message"(w15) -> ()
    }
    frame #2 {
      # "Initialisation des références"
      n147 = disable-structure shown="Disabled" {
        frame Disabled {
          n148 = stacked-sequence {
            frame #0 {
              # "Initialisation references attenuateurs"
              n149 = local read "Nom de base du fichier de références atténuateurs"() -> (w286:string)
              n150 = local read "Adresse des fichiers de référence"() -> (w285:string)
              n151 = for {
                N: 3 -> [_]
                tunnel: w285 -> [w290]
                tunnel: w286 -> [w291]
                i -> [w302]
                # "Lecture des positions de référence : 1 fichier par atténuateur"
                # "Passe l'erreur\nsi le fichier existe\nou si erreur autre que\nle fichier n'existe pas"
                n152 = Increment(x=w302) -> (x+1=w288:i32)
                n153 = Number To Decimal String(number=w288) -> (decimal integer string=w301:string)  [unwired: 1 in]
                n154 = Concatenate Strings(w290, "\\", w291, w301, ".txt" ("string")) -> (w299:string)
                n155 = Build Path(name or relative path=w299) -> (appended path=w295:path)  [unwired: 1 in]
                n156 = Open/Create/Replace File(file path (use dialog)=w295, operation (0:open)=T6."open") -> (refnum out=w293:refnum<file>, error out=w292:errorcluster)  [unwired: 4 in, 1 out]
                n157 = Unbundle By Name(w292) -> ("code"=w294:i32)
                n158 = Equal?(x=w294, y=7) -> (x = y?=w296:bool)
                n159 = case shown="False" w296 {
                  tunnel: w295 -> [_ w318]
                  tunnel: w294 -> [w307 _]
                  tunnel: w293 -> [w304 _]
                  tunnel: w292 -> [w303 _]
                  frame False {
                    n160 = Equal?(x=w307, y=0) -> (x = y?=w305:bool)
                    n161 = case shown="True" w305 {
                      tunnel: w304 -> [_ w311]
                      tunnel: w303 -> [_ w310]
                      frame False {
                      }
                      frame True {
                        # "Si le fichier existe, lit les références"
                        # "Boucle sur les 4 références"
                        n162 = for {
                          N: 4 -> [_]
                          shift-right: [w315] -> w309
                          shift-left: w311 -> [w317]
                          tunnel: w310 -> [w316]
                          tunnel: [w313] -> w308 mode=indexing
                          n163 = Scan From String("%s\\t %d " ("format string"), w317, w316) -> (w315:refnum<file>, output 2=w313:i32)  [unwired: 3 in, 1 out]
                        }
                        n164 = Close File(refnum=w309) -> ()  [unwired: 1 in, 2 out]
                        n165 = property on="Positions de référence" class="Arr (strict)"("Value"=w308) -> ()  [unwired: 2 in, 2 out]
                      }
                    }
                  }
                  frame True {
                    # "Si le fichier n'existe pas (erreur 7), crée le fichier de références"
                    n166 = stacked-sequence {
                      seq-local: [w320 _ _] -> [_ w323 _]
                      seq-local: [w319 _ _] -> [_ _ _]
                      seq-local: [_ w324 _] -> [_ _ w336]
                      tunnel: w318 -> [w322 _ _]
                      frame #0 {
                        n167 = Open/Create/Replace File(file path (use dialog)=w322, operation (0:open)=T6."create") -> (refnum out=w320:refnum<file>, error out=w319:errorcluster)  [unwired: 4 in, 1 out]
                      }
                      frame #1 {
                        # "Boucle sur les 3 références"
                        n168 = for {
                          N: 3 -> [_]
                          shift-right: [w334] -> w324
                          shift-left: w323 -> [w335]
                          i -> [w333]
                          n169 = Increment(x=w333) -> (x+1=w326:i32)
                          n170 = Number To Decimal String(number=w326) -> (decimal integer string=w332:string)  [unwired: 1 in]
                          n171 = Concatenate Strings("Référence", w332, "\t") -> (w330:string)
                          n172 = Format Into String(initial string=w335, w330, 0, "\r\n") -> (resulting string=w334:refnum<file>)  [unwired: 2 in, 1 out]
                        }
                      }
                      frame #2 {
                        n173 = Close File(refnum=w336) -> ()  [unwired: 1 in, 2 out]
                      }
                    }
                  }
                }
              }
            }
          }
        }
        frame Enabled {
        }
      }
    }
    frame #3 {
      n174 = control-ref of="Axe1_PositionTheorique 2"() -> (w345:refnum<vi>)
      n175 = control-ref of="Axe2_PositionTheorique 2"() -> (w344:refnum<vi>)
      n176 = control-ref of="Axe3_PositionTheorique 2"() -> (w343:refnum<vi>)
      n177 = control-ref of="Axe4_PositionTheorique 2"() -> (w339:refnum<vi>)
      n178 = control-ref of="Axe5_PositionTheorique 2"() -> (w338:refnum<vi>)
      n179 = control-ref of="Axe6_PositionTheorique 2"() -> (w337:refnum<vi>)
      n180 = property on="Property Node" class="DigNum (strict)"(reference=w339, "Visible"=FALSE) -> ()  [unwired: 1 in, 2 out]
      n181 = property on="Property Node" class="DigNum (strict)"(reference=w345, "Visible"=TRUE) -> ()  [unwired: 1 in, 2 out]
      n182 = property on="Property Node" class="DigNum (strict)"(reference=w344, "Visible"=FALSE) -> ()  [unwired: 1 in, 2 out]
      n183 = property on="Property Node" class="DigNum (strict)"(reference=w343, "Visible"=FALSE) -> ()  [unwired: 1 in, 2 out]
      n184 = property on="Property Node" class="DigNum (strict)"(reference=w338, "Visible"=FALSE) -> ()  [unwired: 1 in, 2 out]
      n185 = property on="Property Node" class="DigNum (strict)"(reference=w337, "Visible"=FALSE) -> ()  [unwired: 1 in, 2 out]
    }
    frame #4 {
      n186 = while {
        stop <- w349 stop-if-true
        n187 = event shown="[14] \"HeNe Switch\": Value Change" {
          selector: _ -> [_ _ _ _ _ _ _ _ _ _ _ _ _ _ _ _ _ _ _ _ _]
          dyn-events: _ -> [_ _ _ _ _ _ _ _ _ _ _ _ _ _ _ _ _ _ _ _ _]
          timeout: _ -> [_ _ _ _ _ _ _ _ _ _ _ _ _ _ _ _ _ _ _ _ _]
          tunnel: [_ _ _ _ _ _ _ _ _ _ _ _ _ _ _ _ _ _ _ w1104 "stop"] -> w349
          event "Att.", "Actif?", "Onglets": Value Change {
            # "Mise à jour de la position à atteindre"
            n188 = event-data() -> ()  [unwired: 1 in, 6 out]
            n189 = local read "Position Atténuateur"() -> (w351:bool[])
            n190 = local read "Inversion butées"() -> (w350:bool[])
            n191 = local read "Att."() -> (w353:bool[])
            n192 = local read "Position Miroir"() -> (w352:bool[])
            n193 = for {
              tunnel: w353 -> [w358] mode=indexing
              tunnel: w352 -> [w354] mode=indexing
              tunnel: w351 -> [w357] mode=indexing
              tunnel: w350 -> [w356] mode=indexing
              i -> [w355]
              n194 = case shown="False" w358 {
                tunnel: w357 -> [_ w382]
                tunnel: w356 -> [w360 w381]
                tunnel: w355 -> [w359 w380]
                tunnel: w354 -> [w361 _]
                frame False {
                  # "Par défaut:\nButée -"
                  # "Si MIROIR"
                  n195 = case shown="False" w361 {
                    tunnel: w360 -> [w363 _]
                    tunnel: w359 -> [w362 w374]
                    frame False {
                      # "Si FAUX utilise la\nBUTEE"
                      n196 = case shown="True" w363 {
                        tunnel: w362 -> [w367 w370]
                        frame False {
                          # "Si butées non inversées : \nutilise butée -"
                          n197 = local read "Position à atteindre"() -> (w366:string[])
                          n198 = Replace Array Subset(array=w366, new element="Butée Négative", index=w367) -> (w364:string[])
                          n199 = local write "Position à atteindre"(w364) -> ()
                        }
                        frame True {
                          # "Si butées inversées : \nutilise butée +"
                          n200 = local read "Position à atteindre"() -> (w371:string[])
                          n201 = Replace Array Subset(array=w371, new element="Butée Positive", index=w370) -> (w368:string[])
                          n202 = local write "Position à atteindre"(w368) -> ()
                        }
                      }
                    }
                    frame True {
                      # "Si VRAI utilise la\nPOSITION de REFERENCE"
                      n203 = local read "Pos. Ref. Miroir"() -> (w378:i32[])
                      n204 = Index Array(array=w378, index=w374) -> (element=w379:i32)
                      n205 = local read "Position à atteindre"() -> (w373:string[])
                      n206 = Number To Decimal String(number=w379) -> (decimal integer string=w376:string)  [unwired: 1 in]
                      n207 = Concatenate Strings("Position de référence = ", w376) -> (w375:string)
                      n208 = Replace Array Subset(array=w373, new element=w375, index=w374) -> (w372:string[])
                      n209 = local write "Position à atteindre"(w372) -> ()
                    }
                  }
                }
                frame True {
                  # "Par défaut:\nButée +"
                  # "Si ATTENUATEUR"
                  n210 = case shown="False" w382 {
                    tunnel: w381 -> [w384 _]
                    tunnel: w380 -> [w383 w394]
                    frame False {
                      # "Si FAUX alors utilise la BUTEE"
                      n211 = case shown="True" w384 {
                        tunnel: w383 -> [w387 w391]
                        frame False {
                          # "SI BUTEE Non INVERSEE :\nattenuateur = butée +"
                          n212 = local read "Position à atteindre"() -> (w388:string[])
                          n213 = Replace Array Subset(array=w388, new element="Butée Positive", index=w387) -> (w385:string[])
                          n214 = local write "Position à atteindre"(w385) -> ()
                        }
                        frame True {
                          # "SI BUTEE INVERSEE :\nattenuateur = butée -"
                          n215 = local read "Position à atteindre"() -> (w392:string[])
                          n216 = Replace Array Subset(array=w392, new element="Butée Négative", index=w391) -> (w389:string[])
                          n217 = local write "Position à atteindre"(w389) -> ()
                        }
                      }
                    }
                    frame True {
                      # "Si VRAI alors utilise la POSITION\nde REFERENCE"
                      n218 = local read "Pos. Ref. Atténuateur"() -> (w395:i32[])
                      n219 = Index Array(array=w395, index=w394) -> (element=w393:i32)
                      n220 = local read "Position à atteindre"() -> (w398:string[])
                      n221 = Number To Decimal String(number=w393) -> (decimal integer string=w399:string)  [unwired: 1 in]
                      n222 = Concatenate Strings("Position de référence = ", w399) -> (w397:string)
                      n223 = Replace Array Subset(array=w398, new element=w397, index=w394) -> (w396:string[])
                      n224 = local write "Position à atteindre"(w396) -> ()
                    }
                  }
                }
              }
            }
          }
          event "HeNe in?": Value Change {
            n225 = event-data() -> ()  [unwired: 1 in, 6 out]
            n226 = property on="Inversion des butées HeNe" class="Bool (strict)"() -> ("Value"=w403:bool)  [unwired: 2 in, 2 out]
            n227 = property on="Position HeNe" class="Bool (strict)"() -> ("Value"=w404:bool)  [unwired: 2 in, 2 out]
            n228 = property on="Position Laser" class="Bool (strict)"() -> ("Value"=w401:bool)  [unwired: 2 in, 2 out]
            n229 = case shown="False" "HeNe in?" {
              tunnel: w404 -> [_ w419]
              tunnel: w403 -> [w407 w418]
              tunnel: [w406 w417] -> w402
              tunnel: w401 -> [w408 _]
              frame False {
                # "FAUX: Laser (Vrai: HeNe)"
                n230 = case shown="True" w408 {
                  tunnel: [w410 w414] -> w406
                  tunnel: w407 -> [w409 _]
                  frame False {
                    # "SI FAUX : en butée"
                    n231 = case shown="False" w409 {
                      tunnel: ["Butée Négative" ("PosAAtt HeNe") "Butée Positive" ("PosAAtt HeNe")] -> w410
                      frame False {
                        # "Sans inversion des butées  Laser butée Négative"
                      }
                      frame True {
                        # "SI inversion des butées alors Laser butée Positive"
                      }
                    }
                  }
                  frame True {
                    # "Si VRAI alors\nen position de référence"
                    n232 = property on="Position de Référence Laser" class="DigNum (strict)"() -> ("Value"=w413:i32)  [unwired: 2 in, 2 out]
                    n233 = Number To Decimal String(number=w413) -> (decimal integer string=w415:string)  [unwired: 1 in]
                    n234 = Concatenate Strings("Position de référence: " ("PosAAtt HeNe"), w415) -> (w414:string)
                  }
                }
              }
              frame True {
                # "VRAI: HeNe (Faux: Laser)"
                n235 = case shown="True" w419 {
                  tunnel: w418 -> [w421 _]
                  tunnel: [w420 w424] -> w417
                  frame False {
                    # "SI FAUX : en butée"
                    n236 = case shown="True" w421 {
                      tunnel: ["Butée Positive" ("PosAAtt HeNe") "Butée Négative" ("PosAAtt HeNe")] -> w420
                      frame False {
                        # "Sans inversion des butées  HeNe butée +"
                      }
                      frame True {
                        # "SI inversion des butées alors HeNe butée -"
                      }
                    }
                  }
                  frame True {
                    # "Si VRAI alors\nen position de référence"
                    n237 = property on="Position de Référence HeNe" class="DigNum (strict)"() -> ("Value"=w427:i32)  [unwired: 2 in, 2 out]
                    n238 = Number To Decimal String(number=w427) -> (decimal integer string=w425:string)  [unwired: 1 in]
                    n239 = Concatenate Strings("Position de référence: " ("PosAAtt HeNe"), w425) -> (w424:string)
                  }
                }
              }
            }
            n240 = property on="PosAAtt HeNe" class="Str"("Value"=w402) -> ()  [unwired: 2 in, 2 out]
          }
          event "Moteur à référencer": Value Change {
            # "Boucle sur les 4 références"
            n241 = event-data() -> ("NewVal"=w429:T5)  [unwired: 1 in, 5 out]
            n242 = case shown="\"HeNe\"" w429 {
              tunnel: [w450 w459 w468 w477 w484 w491] -> w428
              frame "Atténuateur 1", Default {
                n243 = property on="Axe2_PositionTheorique 2" class="DigNum (strict)"("Visible"=FALSE) -> ()  [unwired: 2 in, 2 out]
                n244 = property on="Axe3_PositionTheorique 2" class="DigNum (strict)"("Visible"=FALSE) -> ()  [unwired: 2 in, 2 out]
                n245 = property on="Axe1_PositionTheorique 2" class="DigNum (strict)"("Visible"=TRUE) -> ()  [unwired: 2 in, 2 out]
                n246 = property on="Axe6_PositionTheorique 2" class="DigNum (strict)"("Visible"=FALSE) -> ()  [unwired: 2 in, 2 out]
                n247 = property on="Axe4_PositionTheorique 2" class="DigNum (strict)"("Visible"=FALSE) -> ()  [unwired: 2 in, 2 out]
                n248 = property on="Axe5_PositionTheorique 2" class="DigNum (strict)"("Visible"=FALSE) -> ()  [unwired: 2 in, 2 out]
                n249 = local read "Nom de base du fichier de références atténuateurs"() -> (w452:string)
                n250 = Concatenate Strings(w452, "1") -> (w450:string)
              }
              frame "Atténuateur 2" {
                n251 = property on="Axe2_PositionTheorique 2" class="DigNum (strict)"("Visible"=TRUE) -> ()  [unwired: 2 in, 2 out]
                n252 = property on="Axe3_PositionTheorique 2" class="DigNum (strict)"("Visible"=FALSE) -> ()  [unwired: 2 in, 2 out]
                n253 = property on="Axe1_PositionTheorique 2" class="DigNum (strict)"("Visible"=FALSE) -> ()  [unwired: 2 in, 2 out]
                n254 = property on="Axe6_PositionTheorique 2" class="DigNum (strict)"("Visible"=FALSE) -> ()  [unwired: 2 in, 2 out]
                n255 = property on="Axe4_PositionTheorique 2" class="DigNum (strict)"("Visible"=FALSE) -> ()  [unwired: 2 in, 2 out]
                n256 = property on="Axe5_PositionTheorique 2" class="DigNum (strict)"("Visible"=FALSE) -> ()  [unwired: 2 in, 2 out]
                n257 = local read "Nom de base du fichier de références atténuateurs"() -> (w460:string)
                n258 = Concatenate Strings(w460, "2") -> (w459:string)
              }
              frame "Atténuateur 3" {
                n259 = property on="Axe2_PositionTheorique 2" class="DigNum (strict)"("Visible"=FALSE) -> ()  [unwired: 2 in, 2 out]
                n260 = property on="Axe3_PositionTheorique 2" class="DigNum (strict)"("Visible"=TRUE) -> ()  [unwired: 2 in, 2 out]
                n261 = property on="Axe1_PositionTheorique 2" class="DigNum (strict)"("Visible"=FALSE) -> ()  [unwired: 2 in, 2 out]
                n262 = property on="Axe6_PositionTheorique 2" class="DigNum (strict)"("Visible"=FALSE) -> ()  [unwired: 2 in, 2 out]
                n263 = property on="Axe4_PositionTheorique 2" class="DigNum (strict)"("Visible"=FALSE) -> ()  [unwired: 2 in, 2 out]
                n264 = property on="Axe5_PositionTheorique 2" class="DigNum (strict)"("Visible"=FALSE) -> ()  [unwired: 2 in, 2 out]
                n265 = local read "Nom de base du fichier de références atténuateurs"() -> (w469:string)
                n266 = Concatenate Strings(w469, "3") -> (w468:string)
              }
              frame "HeNe" {
                n267 = property on="Axe2_PositionTheorique 2" class="DigNum (strict)"("Visible"=FALSE) -> ()  [unwired: 2 in, 2 out]
                n268 = property on="Axe3_PositionTheorique 2" class="DigNum (strict)"("Visible"=FALSE) -> ()  [unwired: 2 in, 2 out]
                n269 = property on="Axe1_PositionTheorique 2" class="DigNum (strict)"("Visible"=FALSE) -> ()  [unwired: 2 in, 2 out]
                n270 = property on="Axe6_PositionTheorique 2" class="DigNum (strict)"("Visible"=FALSE) -> ()  [unwired: 2 in, 2 out]
                n271 = property on="Axe4_PositionTheorique 2" class="DigNum (strict)"("Visible"=TRUE) -> ()  [unwired: 2 in, 2 out]
                n272 = property on="Axe5_PositionTheorique 2" class="DigNum (strict)"("Visible"=FALSE) -> ()  [unwired: 2 in, 2 out]
                n273 = local read "Nom de base du fichier de référence HeNe"() -> (w477:string)
              }
              frame "Miroir Troué" {
                n274 = property on="Axe2_PositionTheorique 2" class="DigNum (strict)"("Visible"=FALSE) -> ()  [unwired: 2 in, 2 out]
                n275 = property on="Axe3_PositionTheorique 2" class="DigNum (strict)"("Visible"=FALSE) -> ()  [unwired: 2 in, 2 out]
                n276 = property on="Axe1_PositionTheorique 2" class="DigNum (strict)"("Visible"=FALSE) -> ()  [unwired: 2 in, 2 out]
                n277 = property on="Axe6_PositionTheorique 2" class="DigNum (strict)"("Visible"=FALSE) -> ()  [unwired: 2 in, 2 out]
                n278 = property on="Axe4_PositionTheorique 2" class="DigNum (strict)"("Visible"=FALSE) -> ()  [unwired: 2 in, 2 out]
                n279 = property on="Axe5_PositionTheorique 2" class="DigNum (strict)"("Visible"=TRUE) -> ()  [unwired: 2 in, 2 out]
                n280 = local read "Nom de base du fichier de référence Miroir Troué"() -> (w484:string)
              }
              frame "Ligne à Retard" {
                n281 = property on="Axe2_PositionTheorique 2" class="DigNum (strict)"("Visible"=FALSE) -> ()  [unwired: 2 in, 2 out]
                n282 = property on="Axe3_PositionTheorique 2" class="DigNum (strict)"("Visible"=FALSE) -> ()  [unwired: 2 in, 2 out]
                n283 = property on="Axe1_PositionTheorique 2" class="DigNum (strict)"("Visible"=FALSE) -> ()  [unwired: 2 in, 2 out]
                n284 = property on="Axe6_PositionTheorique 2" class="DigNum (strict)"("Visible"=TRUE) -> ()  [unwired: 2 in, 2 out]
                n285 = property on="Axe4_PositionTheorique 2" class="DigNum (strict)"("Visible"=FALSE) -> ()  [unwired: 2 in, 2 out]
                n286 = property on="Axe5_PositionTheorique 2" class="DigNum (strict)"("Visible"=FALSE) -> ()  [unwired: 2 in, 2 out]
                n287 = local read "Nom de base du fichier de référence Ligne à Retard"() -> (w491:string)
              }
            }
            n288 = local read "Adresse des fichiers de référence"() -> (w437:string)
            n289 = Concatenate Strings(w437, "\\", w428, ".txt") -> (w440:string)
            n290 = Build Path(name or relative path=w440) -> (appended path=w439:path)  [unwired: 1 in]
            n291 = Open/Create/Replace File(file path (use dialog)=w439, operation (0:open)=T6."open") -> (refnum out=w435:refnum<file>, error out=w436:errorcluster)  [unwired: 4 in, 1 out]
            n292 = for {
              N: 4 -> [_]
              shift-right: [w448] -> w431
              shift-left: w435 -> [w449]
              tunnel: [w445] -> w433 mode=indexing
              tunnel: [w444] -> w432 mode=indexing
              shift-right: [w443] -> w430
              shift-left: w436 -> [w446]
              n293 = Scan From String("%s\\t %d " ("format string"), w449, w446) -> (w448:refnum<file>, w443:errorcluster, output 1=w445:string, output 2=w444:i32)  [unwired: 2 in]
            }
            n294 = local write "Positions de référence"(w432) -> ()
            n295 = local write "Libellés pos. de référence"(w433) -> ()
            n296 = Close File(refnum=w431, error in=w430) -> ()  [unwired: 2 out]
          }
          event "Inc -": Value Change {
            w509 = u16 0 items=["Mouvement Relatif"=1, "Mouvement Absolu"=0] ("Mouvement Absolu/Relatif")
            w513 = T7 2 items=["Mouvement Simple"=1, "Aller vers Cote"=2, "Va vers position de référence"=3] ("Type de mouvement")
            n297 = event-data() -> ()  [unwired: 1 in, 6 out]
            n298 = property on="Moteur à déplacer" class="Enum (strict)"() -> ("Value"=w511:T3)  [unwired: 2 in, 2 out]
            n299 = case shown="\"HeNe\"" w511 {
              tunnel: [u32 1 ("Numéro d'Axe") u32 2 ("Numéro d'Axe") u32 3 ("Numéro d'Axe") u32 4 ("Numéro d'Axe") u32 5 ("Numéro d'Axe") u32 6 ("Numéro d'Axe")] -> w510
              tunnel: [w516 w518 w521 w524 w527 w530] -> w499
              tunnel: [w515 w519 w522 w525 w528 w531] -> w505
              frame "Atténuateur 1", Default {
                n300 = shared-variable "My Computer\\OPCLib.lvlib\\Axe1_PositionTheorique"() -> (w516:i32)  [unwired: 1 in, 1 out]
                n301 = local read "Attenuateurs\n(µm/pas)"() -> (w515:dbl)
              }
              frame "Atténuateur 2" {
                n302 = shared-variable "My Computer\\OPCLib.lvlib\\Axe2_PositionTheorique"() -> (w518:i32)  [unwired: 1 in, 1 out]
                n303 = local read "Attenuateurs\n(µm/pas)"() -> (w519:dbl)
              }
              frame "Atténuateur 3" {
                n304 = shared-variable "My Computer\\OPCLib.lvlib\\Axe3_PositionTheorique"() -> (w521:i32)  [unwired: 1 in, 1 out]
                n305 = local read "Attenuateurs\n(µm/pas)"() -> (w522:dbl)
              }
              frame "HeNe" {
                n306 = shared-variable "My Computer\\OPCLib.lvlib\\Axe4_PositionTheorique"() -> (w524:i32)  [unwired: 1 in, 1 out]
                n307 = local read "HeNe\n(µm/pas)"() -> (w525:dbl)
              }
              frame "Miroir Troué" {
                n308 = shared-variable "My Computer\\OPCLib.lvlib\\Axe5_PositionTheorique"() -> (w527:i32)  [unwired: 1 in, 1 out]
                n309 = local read "MT (µm/pas)"() -> (w528:dbl)
              }
              frame "Delay Line" {
                n310 = shared-variable "My Computer\\OPCLib.lvlib\\Axe6_PositionTheorique"() -> (w530:i32)  [unwired: 1 in, 1 out]
                n311 = local read "LR (µm/pas)"() -> (w531:dbl)
              }
            }
            n312 = local read "Adresse du PilMOT"() -> (w514:string)
            n313 = property on="Increment (mm)" class="DigNum (strict)"() -> ("Value"=w508:dbl)  [unwired: 2 in, 2 out]
            n314 = call "FetchAxisSharedVars.vi"("Numéro d'Axe"=w510, "PilMOT Address"=w514) -> ("error out"=w501:errorcluster, "Sortie Variables d'Axes"=w502:T8)  [unwired: 8 in]
            n315 = Divide(x=w508, y=1000.0) -> (x/y=w506:dbl)
            n316 = Divide(x=w506, y=w505) -> (x/y=w504:dbl)
            n317 = Round To Nearest(number=w504) -> (nearest integer value=w503:dbl)
            n318 = To Long Integer(number=w503) -> (32bit integer=w500:i32)
            n319 = Subtract(x=w499, y=w500) -> (x-y=w498:i32)
            n320 = call "MovePilMot.vi"("Variables d'Axes"=w502, "Cote à atteindre"=w498, "error in (no error)"=w501, "Type de mouvement"=w513, "Mouvement Absolu/Relatif"=w509) -> ("error out"=w512:errorcluster)  [unwired: 10 in]
            n321 = local write "error out"(w512) -> ()
          }
          event "Inc +": Value Change {
            w544 = u16 0 items=["Mouvement Relatif"=1, "Mouvement Absolu"=0] ("Mouvement Absolu/Relatif")
            w548 = T7 2 items=["Mouvement Simple"=1, "Aller vers Cote"=2, "Va vers position de référence"=3] ("Type de mouvement")
            n322 = event-data() -> ()  [unwired: 1 in, 6 out]
            n323 = property on="Moteur à déplacer" class="Enum (strict)"() -> ("Value"=w546:T3)  [unwired: 2 in, 2 out]
            n324 = case shown="\"HeNe\"" w546 {
              tunnel: [u32 1 ("Numéro d'Axe") u32 2 ("Numéro d'Axe") u32 3 ("Numéro d'Axe") u32 4 ("Numéro d'Axe") u32 5 ("Numéro d'Axe") u32 6 ("Numéro d'Axe")] -> w545
              tunnel: [w551 w553 w556 w559 w562 w565] -> w534
              tunnel: [w550 w554 w557 w560 w563 w566] -> w540
              frame "Atténuateur 1", Default {
                n325 = shared-variable "My Computer\\OPCLib.lvlib\\Axe1_PositionTheorique"() -> (w551:i32)  [unwired: 1 in, 1 out]
                n326 = local read "Attenuateurs\n(µm/pas)"() -> (w550:dbl)
              }
              frame "Atténuateur 2" {
                n327 = shared-variable "My Computer\\OPCLib.lvlib\\Axe2_PositionTheorique"() -> (w553:i32)  [unwired: 1 in, 1 out]
                n328 = local read "Attenuateurs\n(µm/pas)"() -> (w554:dbl)
              }
              frame "Atténuateur 3" {
                n329 = shared-variable "My Computer\\OPCLib.lvlib\\Axe3_PositionTheorique"() -> (w556:i32)  [unwired: 1 in, 1 out]
                n330 = local read "Attenuateurs\n(µm/pas)"() -> (w557:dbl)
              }
              frame "HeNe" {
                n331 = shared-variable "My Computer\\OPCLib.lvlib\\Axe4_PositionTheorique"() -> (w559:i32)  [unwired: 1 in, 1 out]
                n332 = local read "HeNe\n(µm/pas)"() -> (w560:dbl)
              }
              frame "Miroir Troué" {
                n333 = shared-variable "My Computer\\OPCLib.lvlib\\Axe5_PositionTheorique"() -> (w562:i32)  [unwired: 1 in, 1 out]
                n334 = local read "MT (µm/pas)"() -> (w563:dbl)
              }
              frame "Delay Line" {
                n335 = shared-variable "My Computer\\OPCLib.lvlib\\Axe6_PositionTheorique"() -> (w565:i32)  [unwired: 1 in, 1 out]
                n336 = local read "LR (µm/pas)"() -> (w566:dbl)
              }
            }
            n337 = local read "Adresse du PilMOT"() -> (w549:string)
            n338 = property on="Increment (mm)" class="DigNum (strict)"() -> ("Value"=w543:dbl)  [unwired: 2 in, 2 out]
            n339 = call "FetchAxisSharedVars.vi"("Numéro d'Axe"=w545, "PilMOT Address"=w549) -> ("error out"=w536:errorcluster, "Sortie Variables d'Axes"=w537:T8)  [unwired: 8 in]
            n340 = Divide(x=w543, y=1000.0) -> (x/y=w541:dbl)
            n341 = Divide(x=w541, y=w540) -> (x/y=w539:dbl)
            n342 = Round To Nearest(number=w539) -> (nearest integer value=w538:dbl)
            n343 = To Long Integer(number=w538) -> (32bit integer=w535:i32)
            n344 = Add(x=w534, y=w535) -> (x+y=w533:i32)
            n345 = call "MovePilMot.vi"("Variables d'Axes"=w537, "Cote à atteindre"=w533, "error in (no error)"=w536, "Type de mouvement"=w548, "Mouvement Absolu/Relatif"=w544) -> ("error out"=w547:errorcluster)  [unwired: 10 in]
            n346 = local write "error out"(w547) -> ()
          }
          event "Set ref", "Go to ref": Value Change {
            # "Réécriture du fichier de références"
            n347 = event-data() -> ()  [unwired: 1 in, 6 out]
            n348 = property on="Moteur à référencer" class="Enum (strict)"() -> ("Value"=w570:T5)  [unwired: 2 in, 2 out]
            n349 = case shown="True" "Set ref" {
              tunnel: w570 -> [_ w574]
              frame False {
              }
              frame True {
                n350 = case shown="\"Atténuateur 1\"..\"Atténuateur 3\"" w574 {
                  tunnel: [w575 w633 w679 w725] -> w573
                  frame "Atténuateur 1".."Atténuateur 3" {
                    n351 = Two Button Dialog(message="Es-tu certain(e) de vouloir remplacer\ncette référence atténuateur?  ", 1:"Non" ("F button name (\"Cancel\")"), 2:"Oui" ("T button name (\"OK\")")) -> (T button?=w576:bool)
                    n352 = case shown="True" w576 {
                      tunnel: ["Canceled by user." w581] -> w575
                      frame False {
                      }
                      frame True {
                        n353 = stacked-sequence {
                          seq-local: [_ w602 _] -> [_ _ w608]
                          seq-local: [w582 _ _] -> [_ w601 _]
                          tunnel: [_ _ w607] -> w581
                          frame #0 {
                            # "ecriture de la nouvelle valeur sur l'interface"
                            n354 = local read "Moteur à référencer"() -> (w588:T5)
                            n355 = case shown="\"Atténuateur 3\"" w588 {
                              tunnel: [w592 w596 w600] -> w583
                              tunnel: [w589 w593 w597] -> w582
                              frame "Atténuateur 1", Default {
                                n356 = local read "Nom de base du fichier de références atténuateurs"() -> (w591:string)
                                n357 = local read "Axe1_PositionTheorique 2"() -> (w592:i32)
                                n358 = Concatenate Strings(w591, "1") -> (w589:string)
                              }
                              frame "Atténuateur 2" {
                                n359 = local read "Nom de base du fichier de références atténuateurs"() -> (w595:string)
                                n360 = local read "Axe2_PositionTheorique 2"() -> (w596:i32)
                                n361 = Concatenate Strings(w595, "2") -> (w593:string)
                              }
                              frame "Atténuateur 3" {
                                n362 = local read "Nom de base du fichier de références atténuateurs"() -> (w599:string)
                                n363 = local read "Axe3_PositionTheorique 2"() -> (w600:i32)
                                n364 = Concatenate Strings(w599, "3") -> (w597:string)
                              }
                            }
                            n365 = local read "Numéro de Pos. Ref."() -> (w586:T4)
                            n366 = To Long Integer(number=w586) -> (32bit integer=w587:i32)
                            n367 = local read "Positions de référence"() -> (w585:i32[])
                            n368 = Replace Array Subset(array=w585, new element=w583, index=w587) -> (w584:i32[])
                            n369 = local write "Positions de référence"(w584) -> ()
                          }
                          frame #1 {
                            # "Construction du chemin d'écriture du fichier"
                            n370 = local read "Adresse des fichiers de référence"() -> (w606:string)
                            n371 = Concatenate Strings(w606, "\\", w601, ".txt") -> (w603:string)
                            n372 = Build Path(name or relative path=w603) -> (appended path=w602:path)  [unwired: 1 in]
                          }
                          frame #2 {
                            n373 = stacked-sequence {
                              seq-local: [w611 _ _] -> [_ w618 _]
                              seq-local: [w610 _ _] -> [_ w617 _]
                              seq-local: [_ w616 _] -> [_ _ w631]
                              seq-local: [_ w615 _] -> [_ _ w632]
                              tunnel: w608 -> [w609 _ _]
                              tunnel: [_ _ w629] -> w607
                              frame #0 {
                                n374 = Open/Create/Replace File(file path (use dialog)=w609, operation (0:open)=T6."open") -> (refnum out=w611:refnum<file>, error out=w610:errorcluster)  [unwired: 4 in, 1 out]
                              }
                              frame #1 {
                                # "Boucle sur les 4 références"
                                n375 = local read "Libellés pos. de référence"() -> (w614:string[])
                                n376 = local read "Positions de référence"() -> (w613:i32[])
                                n377 = for {
                                N: 4 -> [_]
                                shift-right: [w627] -> w616
                                shift-left: w618 -> [w628]
                                shift-right: [w623] -> w615
                                shift-left: w617 -> [w624]
                                tunnel: w614 -> [w622] mode=indexing
                                tunnel: w613 -> [w621] mode=indexing
                                n378 = Concatenate Strings(w622, "\t") -> (w626:string)
                                n379 = Format Into String(initial string=w628, error in=w624, w626, w621, "\r\n") -> (resulting string=w627:refnum<file>, error out=w623:errorcluster)  [unwired: 1 in]
                                }
                              }
                              frame #2 {
                                n380 = Close File(refnum=w631, error in=w632) -> (error out=w630:errorcluster)  [unwired: 1 out]
                                n381 = Unbundle By Name(w630) -> ("source"=w629:string)
                                n382 = local write "error out"(w630) -> ()
                              }
                            }
                          }
                        }
                      }
                    }
                  }
                  frame "HeNe" {
                    n383 = stacked-sequence {
                      seq-local: [_ w639 _ _] -> [_ _ _ w650]
                      seq-local: [_ _ w643 _] -> [_ _ _ w651]
                      tunnel: [_ _ _ w649] -> w633
                      frame #0 {
                        # "UNFINISHED!!!!"
                        # "ecriture de la nouvelle valeur sur l'interface"
                        n384 = local read "Axe4_PositionTheorique 2"() -> (w634:i32)
                        n385 = local read "Numéro de Pos. Ref."() -> (w637:T4)
                        n386 = local read "Positions de référence"() -> (w636:i32[])
                        n387 = To Long Integer(number=w637) -> (32bit integer=w638:i32)
                        n388 = Replace Array Subset(array=w636, new element=w634, index=w638) -> (w635:i32[])
                        n389 = local write "Positions de référence"(w635) -> ()
                      }
                      frame #1 {
                        n390 = Two Button Dialog(message="Es-tu certain(e) de vouloir remplacer\ncette référence pour l'HeNe?  ", 1:"Non" ("F button name (\"Cancel\")"), 2:"Oui" ("T button name (\"OK\")")) -> (T button?=w639:bool)
                      }
                      frame #2 {
                        # "Construction du chemin d'écriture du fichier"
                        n391 = local read "Nom de base du fichier de référence HeNe"() -> (w646:string)
                        n392 = local read "Adresse des fichiers de référence"() -> (w648:string)
                        n393 = Concatenate Strings(w648, "\\", w646, ".txt") -> (w644:string)
                        n394 = Build Path(name or relative path=w644) -> (appended path=w643:path)  [unwired: 1 in]
                      }
                      frame #3 {
                        n395 = case shown="False" w650 {
                          tunnel: w651 -> [_ w655]
                          tunnel: ["Canceled by user." w653] -> w649
                          frame False {
                          }
                          frame True {
                            n396 = stacked-sequence {
                              seq-local: [w658 _ _] -> [_ w665 _]
                              seq-local: [w657 _ _] -> [_ w664 _]
                              seq-local: [_ w663 _] -> [_ _ w677]
                              seq-local: [_ w662 _] -> [_ _ w678]
                              tunnel: w655 -> [w656 _ _]
                              tunnel: [_ _ w676] -> w654
                              frame #0 {
                                n397 = Open/Create/Replace File(file path (use dialog)=w656, operation (0:open)=T6."open or create") -> (refnum out=w658:refnum<file>, error out=w657:errorcluster)  [unwired: 4 in, 1 out]
                              }
                              frame #1 {
                                # "Boucle sur les 4 références"
                                n398 = local read "Libellés pos. de référence"() -> (w661:string[])
                                n399 = local read "Positions de référence"() -> (w660:i32[])
                                n400 = for {
                                N: 4 -> [_]
                                shift-right: [w674] -> w663
                                shift-left: w665 -> [w675]
                                shift-right: [w670] -> w662
                                shift-left: w664 -> [w671]
                                tunnel: w661 -> [w669] mode=indexing
                                tunnel: w660 -> [w668] mode=indexing
                                n401 = Concatenate Strings(w669, "\t") -> (w673:string)
                                n402 = Format Into String(initial string=w675, error in=w671, w673, w668, "\r\n") -> (resulting string=w674:refnum<file>, error out=w670:errorcluster)  [unwired: 1 in]
                                }
                              }
                              frame #2 {
                                n403 = Close File(refnum=w677, error in=w678) -> (error out=w676:errorcluster)  [unwired: 1 out]
                                n404 = local write "error out"(w676) -> ()
                              }
                            }
                            n405 = Unbundle By Name(w654) -> ("source"=w653:string)
                          }
                        }
                      }
                    }
                  }
                  frame "Miroir Troué" {
                    n406 = stacked-sequence {
                      seq-local: [_ w685 _ _] -> [_ _ _ w696]
                      seq-local: [_ _ w689 _] -> [_ _ _ w697]
                      tunnel: [_ _ _ w695] -> w679
                      frame #0 {
                        # "UNFINISHED!!!!"
                        # "ecriture de la nouvelle valeur sur l'interface"
                        n407 = local read "Axe5_PositionTheorique 2"() -> (w680:i32)
                        n408 = local read "Numéro de Pos. Ref."() -> (w683:T4)
                        n409 = local read "Positions de référence"() -> (w682:i32[])
                        n410 = To Long Integer(number=w683) -> (32bit integer=w684:i32)
                        n411 = Replace Array Subset(array=w682, new element=w680, index=w684) -> (w681:i32[])
                        n412 = local write "Positions de référence"(w681) -> ()
                      }
                      frame #1 {
                        n413 = Two Button Dialog(message="Es-tu certain(e) de vouloir remplacer\ncette référence pour le miroir troué?  ", 1:"Non" ("F button name (\"Cancel\")"), 2:"Oui" ("T button name (\"OK\")")) -> (T button?=w685:bool)
                      }
                      frame #2 {
                        # "Construction du chemin d'écriture du fichier"
                        n414 = local read "Nom de base du fichier de référence Miroir Troué"() -> (w692:string)
                        n415 = local read "Adresse des fichiers de référence"() -> (w694:string)
                        n416 = Concatenate Strings(w694, "\\", w692, ".txt") -> (w690:string)
                        n417 = Build Path(name or relative path=w690) -> (appended path=w689:path)  [unwired: 1 in]
                      }
                      frame #3 {
                        n418 = case shown="True" w696 {
                          tunnel: w697 -> [_ w701]
                          tunnel: ["Canceled by user." ("Message") w699] -> w695
                          frame False {
                          }
                          frame True {
                            n419 = stacked-sequence {
                              seq-local: [w704 _ _] -> [_ w711 _]
                              seq-local: [w703 _ _] -> [_ w710 _]
                              seq-local: [_ w709 _] -> [_ _ w723]
                              seq-local: [_ w708 _] -> [_ _ w724]
                              tunnel: w701 -> [w702 _ _]
                              tunnel: [_ _ w722] -> w700
                              frame #0 {
                                n420 = Open/Create/Replace File(file path (use dialog)=w702, operation (0:open)=T6."open or create") -> (refnum out=w704:refnum<file>, error out=w703:errorcluster)  [unwired: 4 in, 1 out]
                              }
                              frame #1 {
                                # "Boucle sur les 4 références"
                                n421 = local read "Libellés pos. de référence"() -> (w707:string[])
                                n422 = local read "Positions de référence"() -> (w706:i32[])
                                n423 = for {
                                N: 4 -> [_]
                                shift-right: [w720] -> w709
                                shift-left: w711 -> [w721]
                                shift-right: [w716] -> w708
                                shift-left: w710 -> [w717]
                                tunnel: w707 -> [w715] mode=indexing
                                tunnel: w706 -> [w714] mode=indexing
                                n424 = Concatenate Strings(w715, "\t") -> (w719:string)
                                n425 = Format Into String(initial string=w721, error in=w717, w719, w714, "\r\n") -> (resulting string=w720:refnum<file>, error out=w716:errorcluster)  [unwired: 1 in]
                                }
                              }
                              frame #2 {
                                n426 = Close File(refnum=w723, error in=w724) -> (error out=w722:errorcluster)  [unwired: 1 out]
                                n427 = local write "error out"(w722) -> ()
                              }
                            }
                            n428 = Unbundle By Name(w700) -> ("source"=w699:string)
                          }
                        }
                      }
                    }
                  }
                  frame "Ligne à Retard" {
                    n429 = stacked-sequence {
                      seq-local: [_ w731 _ _] -> [_ _ _ w742]
                      seq-local: [_ _ w735 _] -> [_ _ _ w743]
                      tunnel: [_ _ _ w741] -> w725
                      frame #0 {
                        # "ecriture de la nouvelle valeur sur l'interface"
                        n430 = local read "Axe6_PositionTheorique 2"() -> (w726:i32)
                        n431 = local read "Numéro de Pos. Ref."() -> (w729:T4)
                        n432 = local read "Positions de référence"() -> (w728:i32[])
                        n433 = To Long Integer(number=w729) -> (32bit integer=w730:i32)
                        n434 = Replace Array Subset(array=w728, new element=w726, index=w730) -> (w727:i32[])
                        n435 = local write "Positions de référence"(w727) -> ()
                      }
                      frame #1 {
                        n436 = Two Button Dialog(message="Es-tu certain(e) de vouloir remplacer\ncette référence pour la ligne à retard?  ", 1:"Non" ("F button name (\"Cancel\")"), 2:"Oui" ("T button name (\"OK\")")) -> (T button?=w731:bool)
                      }
                      frame #2 {
                        # "Construction du chemin d'écriture du fichier"
                        n437 = local read "Nom de base du fichier de référence Ligne à Retard"() -> (w738:string)
                        n438 = local read "Adresse des fichiers de référence"() -> (w740:string)
                        n439 = Concatenate Strings(w740, "\\", w738, ".txt") -> (w736:string)
                        n440 = Build Path(name or relative path=w736) -> (appended path=w735:path)  [unwired: 1 in]
                      }
                      frame #3 {
                        n441 = case shown="True" w742 {
                          tunnel: w743 -> [_ w747]
                          tunnel: ["Canceled by user." w745] -> w741
                          frame False {
                          }
                          frame True {
                            n442 = stacked-sequence {
                              seq-local: [w750 _ _] -> [_ w757 _]
                              seq-local: [w749 _ _] -> [_ w756 _]
                              seq-local: [_ w755 _] -> [_ _ w769]
                              seq-local: [_ w754 _] -> [_ _ w770]
                              tunnel: w747 -> [w748 _ _]
                              tunnel: [_ _ w768] -> w746
                              frame #0 {
                                n443 = Open/Create/Replace File(file path (use dialog)=w748, operation (0:open)=T6."open or create") -> (refnum out=w750:refnum<file>, error out=w749:errorcluster)  [unwired: 4 in, 1 out]
                              }
                              frame #1 {
                                # "Boucle sur les 4 références"
                                n444 = local read "Libellés pos. de référence"() -> (w753:string[])
                                n445 = local read "Positions de référence"() -> (w752:i32[])
                                n446 = for {
                                N: 4 -> [_]
                                shift-right: [w766] -> w755
                                shift-left: w757 -> [w767]
                                shift-right: [w762] -> w754
                                shift-left: w756 -> [w763]
                                tunnel: w753 -> [w761] mode=indexing
                                tunnel: w752 -> [w760] mode=indexing
                                n447 = Concatenate Strings(w761, "\t") -> (w765:string)
                                n448 = Format Into String(initial string=w767, error in=w763, w765, w760, "\r\n") -> (resulting string=w766:refnum<file>, error out=w762:errorcluster)  [unwired: 1 in]
                                }
                              }
                              frame #2 {
                                n449 = Close File(refnum=w769, error in=w770) -> (error out=w768:errorcluster)  [unwired: 1 out]
                                n450 = local write "error out"(w768) -> ()
                              }
                            }
                            n451 = Unbundle By Name(w746) -> ("source"=w745:string)
                          }
                        }
                      }
                    }
                  }
                }
                n452 = property on="Message" class="Str"("Value"=w573) -> ()  [unwired: 2 in, 2 out]
              }
            }
            n453 = case shown="True" "Go to ref" {
              frame False {
              }
              frame True {
                w772 = u16 0 items=["Mouvement Relatif"=1, "Mouvement Absolu"=0] ("Mouvement Absolu/Relatif")
                w773 = T7 2 items=["Mouvement Simple"=1, "Aller vers Cote"=2, "Va vers position de référence"=3] ("Type de mouvement")
                n454 = local read "Numéro de Pos. Ref."() -> (w776:T4)
                n455 = local read "Positions de référence"() -> (w777:i32[])
                n456 = local read "Moteur à référencer"() -> (w782:T5)
                n457 = local read "Adresse du PilMOT"() -> (w783:string)
                n458 = To Long Integer(number=w776) -> (32bit integer=w775:i32)
                n459 = Increment(x=w782) -> (x+1=w771:T5)
                n460 = Index Array(array=w777, index=w775) -> (element=w774:i32)
                n461 = To Unsigned Long Integer(number=w771) -> (unsigned 32bit integer=w781:u32)
                n462 = call "FetchAxisSharedVars.vi"("Numéro d'Axe"=w781, "PilMOT Address"=w783) -> ("error out"=w779:errorcluster, "Sortie Variables d'Axes"=w778:T8)  [unwired: 8 in]
                n463 = call "MovePilMot.vi"("Variables d'Axes"=w778, "Cote à atteindre"=w774, "error in (no error)"=w779, "Type de mouvement"=w773, "Mouvement Absolu/Relatif"=w772) -> ("error out"=w780:errorcluster)  [unwired: 10 in]
                n464 = local write "error out"(w780) -> ()
              }
            }
            n465 = local read "Moteur à référencer"() -> (w568:T5)
            n466 = Increment(x=w568) -> (x+1=w569:T5)
            n467 = Number To Decimal String(number=w569) -> ()  [unwired: 1 in, 1 out]
          }
          event "Déplacer +", "Deplacer -", "Butée -", "Butée +", "Origine ici", "Ref. Tab Déplacer +", "Ref. Tab Deplacer -", "Ref. Tab Butée +", "Ref. Tab Butée -", "Ref. Tab. Origine ici": Value Change {
            w823 = T7 1 items=["Mouvement Simple"=1, "Aller vers Cote"=2, "Va vers position de référence"=3] ("Type de mouvement")
            # "Ordre UC Origine"
            # "Déplacements manuels"
            # "Ordre UC mvt +"
            # "Ordre UC mvt -"
            # "Ordre UC butée +"
            # "Ordre UC butée -"
            n468 = event-data() -> ()  [unwired: 1 in, 6 out]
            n469 = local read "Onglets"() -> (w785:T1)
            n470 = Or(x="Ref. Tab. Origine ici", y="Origine ici") -> (x .or. y?=w787:bool)
            n471 = case shown="\"Déplacement manuel, positions mir./att.\"" w785 {
              tunnel: [w828 w829 _ _] -> w784
              frame "Déplacement manuel, positions mir./att." {
                n472 = local read "Moteur à déplacer"() -> (w828:T3)
              }
              frame "Positions de référence" {
                n473 = local read "Moteur à référencer"() -> (w829:T5)
              }
              frame "Configuration   " {
              }
              frame "Attenuation/Déplacements   " {
              }
            }
            n474 = Or(x="Ref. Tab Deplacer -", y="Deplacer -") -> (x .or. y?=w798:bool)
            n475 = Or(x="Ref. Tab Butée +", y="Butée +") -> (x .or. y?=w793:bool)
            n476 = Or(x="Ref. Tab Butée -", y="Butée -") -> (x .or. y?=w792:bool)
            n477 = Or(x="Ref. Tab Déplacer +", y="Déplacer +") -> (x .or. y?=w801:bool)
            n478 = Boolean To (0,1)(Boolean=w787) -> (0, 1=w807:i16)
            n479 = Boolean To (0,1)(Boolean=w801) -> (0, 1=w822:i16)
            n480 = Boolean To (0,1)(Boolean=w798) -> (0, 1=w820:i16)
            n481 = Boolean To (0,1)(Boolean=w793) -> (0, 1=w818:i16)
            n482 = Boolean To (0,1)(Boolean=w792) -> (0, 1=w816:i16)
            n483 = Multiply(x=w807, y=u16 2) -> (x*y=w805:u16)
            n484 = Multiply(x=w822, y=u16 16 ("Ordre UC")) -> (x*y=w814:u16)
            n485 = Multiply(x=w820, y=u16 32 ("Ordre UC")) -> (x*y=w813:u16)
            n486 = Multiply(x=w816, y=u16 128 ("Ordre UC")) -> (x*y=w811:u16)
            n487 = Multiply(x=w818, y=u16 64 ("Ordre UC")) -> (x*y=w812:u16)
            n488 = Select(t=u16 16 ("y"), s=w787, f=u16 0) -> (s? t:f=w802:u16)
            n489 = To Unsigned Long Integer(number=w784) -> (unsigned 32bit integer=w786:u32)
            n490 = local read "Adresse du PilMOT"() -> (w825:string)
            n491 = Add(x=w786, y=u32 1) -> (x+y=w827:u32)
            n492 = Compound Arithmetic op=ADD(w814, w813, w812, w811, w805) -> (w809:u16)
            n493 = call "FetchAxisSharedVars.vi"("Numéro d'Axe"=w827, "PilMOT Address"=w825) -> ("error out"=w810:errorcluster, "Sortie Variables d'Axes"=w824:T8)  [unwired: 8 in]
            n494 = call "MovePilMot.vi"("Ordre UC"=w809, "Variables d'Axes"=w824, "error in (no error)"=w810, "Type de mouvement"=w823, "Ordre Bloc"=w802) -> ("error out"=w808:errorcluster)  [unwired: 10 in]
            n495 = local write "error out"(w808) -> ()
          }
          event "Set Miroir": Value Change {
            n496 = event-data() -> ()  [unwired: 1 in, 1 out]
            n497 = local read "Atténuateur  à référencer"() -> (w832:T2)
            n498 = case shown="\"Atténuateur 3\"" w832 {
              tunnel: [w834 w835 w836] -> w831
              frame "Atténuateur 1", Default {
                n499 = local read "Axe1_PositionTheorique"() -> (w834:i32)
              }
              frame "Atténuateur 2" {
                n500 = local read "Axe2_PositionTheorique"() -> (w835:i32)
              }
              frame "Atténuateur 3" {
                n501 = local read "Axe3_PositionTheorique"() -> (w836:i32)
              }
            }
            n502 = local read "Pos. Ref. Miroir"() -> (w833:i32[])
            n503 = Replace Array Subset(array=w833, new element=w831, index=w832) -> (w830:i32[])
            n504 = local write "Pos. Ref. Miroir"(w830) -> ()
          }
          event "LR Deplacer": Value Change {
            w845 = T7 2 items=["Mouvement Simple"=1, "Aller vers Cote"=2, "Va vers position de référence"=3] ("Type de mouvement")
            n505 = event-data() -> ()  [unwired: 1 in, 6 out]
            n506 = local read "LR (µm/pas)"() -> (w841:dbl)
            n507 = Divide(x="LR Déplacement (µm)", y=w841) -> (x/y=w839:dbl)
            n508 = Round To Nearest(number=w839) -> (nearest integer value=w838:dbl)
            n509 = case shown="\"Absolu\", Default" "LR Type Mouvement" {
              tunnel: [w849 w850] -> w843
              frame "Absolu", Default {
                w849 = u16 0 items=["Mouvement Relatif"=1, "Mouvement Absolu"=0] ("Mouvement Absolu/Relatif")
              }
              frame "Relatif" {
                w850 = u16 1 items=["Mouvement Relatif"=1, "Mouvement Absolu"=0] ("Mouvement Absolu/Relatif")
              }
            }
            n510 = To Long Integer(number=w838) -> (32bit integer=w837:i32)
            n511 = local read "Adresse du PilMOT"() -> (w848:string)
            n512 = call "FetchAxisSharedVars.vi"("Numéro d'Axe"=u32 6, "PilMOT Address"=w848) -> ("Sortie Variables d'Axes"=w846:T8)  [unwired: 8 in, 1 out]
            n513 = call "MovePilMot.vi"("Variables d'Axes"=w846, "Cote à atteindre"=w837, "Type de mouvement"=w845, "Mouvement Absolu/Relatif"=w843) -> ("error out"=w844:errorcluster)  [unwired: 11 in]
            n514 = local write "error out"(w844) -> ()
          }
          event "MT Deplacer": Value Change {
            w859 = T7 2 items=["Mouvement Simple"=1, "Aller vers Cote"=2, "Va vers position de référence"=3] ("Type de mouvement")
            n515 = event-data() -> ()  [unwired: 1 in, 6 out]
            n516 = case shown="\"Relatif\"" "MT Type Mouvement" {
              tunnel: [w863 w864] -> w856
              frame "Absolu", Default {
                w863 = u16 0 items=["Mouvement Relatif"=1, "Mouvement Absolu"=0] ("Mouvement Absolu/Relatif")
              }
              frame "Relatif" {
                w864 = u16 1 items=["Mouvement Relatif"=1, "Mouvement Absolu"=0] ("Mouvement Absolu/Relatif")
              }
            }
            n517 = local read "MT (µm/pas)"() -> (w853:dbl)
            n518 = local read "Adresse du PilMOT"() -> (w862:string)
            n519 = Divide(x="MT Déplacement (µm)", y=w853) -> (x/y=w855:dbl)
            n520 = Round To Nearest(number=w855) -> (nearest integer value=w854:dbl)
            n521 = To Long Integer(number=w854) -> (32bit integer=w851:i32)
            n522 = call "FetchAxisSharedVars.vi"("Numéro d'Axe"=u32 5, "PilMOT Address"=w862) -> ("Sortie Variables d'Axes"=w860:T8)  [unwired: 8 in, 1 out]
            n523 = call "MovePilMot.vi"("Variables d'Axes"=w860, "Cote à atteindre"=w851, "Type de mouvement"=w859, "Mouvement Absolu/Relatif"=w856) -> ("error out"=w858:errorcluster)  [unwired: 11 in]
            n524 = local write "error out"(w858) -> ()
          }
          event "Set Atténuateur": Value Change {
            n525 = event-data() -> ()  [unwired: 1 in, 6 out]
            n526 = local read "Atténuateur  à référencer"() -> (w868:T2)
            n527 = case shown="\"Atténuateur 3\"" w868 {
              tunnel: [w869 w870 w871] -> w867
              frame "Atténuateur 1", Default {
                n528 = local read "Axe1_PositionTheorique"() -> (w869:i32)
              }
              frame "Atténuateur 2" {
                n529 = local read "Axe2_PositionTheorique"() -> (w870:i32)
              }
              frame "Atténuateur 3" {
                n530 = local read "Axe3_PositionTheorique"() -> (w871:i32)
              }
            }
            n531 = local read "Pos. Ref. Atténuateur"() -> (w866:i32[])
            n532 = Replace Array Subset(array=w866, new element=w867, index=w868) -> (w865:i32[])
            n533 = local write "Pos. Ref. Atténuateur"(w865) -> ()
          }
          event "Set HeNe": Value Change {
            n534 = event-data() -> ()  [unwired: 1 in, 6 out]
            n535 = local read "Axe4_PositionTheorique"() -> (w872:i32)
            n536 = property on="Position de Référence HeNe" class="DigNum (strict)"("Value"=w872) -> ()  [unwired: 2 in, 2 out]
          }
          event "Set Laser": Value Change {
            n537 = event-data() -> ()  [unwired: 1 in, 6 out]
            n538 = local read "Axe4_PositionTheorique"() -> (w873:i32)
            n539 = property on="Position de Référence Laser" class="DigNum (strict)"("Value"=w873) -> ()  [unwired: 2 in, 2 out]
          }
          event "Attenuer": Value Change {
            # "inversion butées"
            # "position mir."
            # "position att."
            n540 = event-data() -> ()  [unwired: 1 in, 6 out]
            n541 = local read "Pos. Ref. Atténuateur"() -> (w878:i32[])
            n542 = local read "Pos. Ref. Miroir"() -> (w879:i32[])
            n543 = local read "Actif?"() -> (w880:bool[])
            n544 = local read "Att."() -> (w883:bool[])
            n545 = local read "error in"() -> (w882:errorcluster)
            n546 = for {
              N: 3 -> [_]
              tunnel: w883 -> [w890] mode=indexing
              shift-right: [w891] -> w881
              shift-left: w882 -> [w892]
              tunnel: w880 -> [w889] mode=indexing
              tunnel: w879 -> [w887] mode=indexing
              tunnel: w878 -> [w888] mode=indexing
              tunnel: "Position Miroir" -> [w886] mode=indexing
              tunnel: "Position Atténuateur" -> [w885] mode=indexing
              tunnel: "Inversion butées" -> [w884] mode=indexing
              i -> [w893]
              # "Boucle sur les 3 axes"
              n547 = case shown="True" w889 {
                tunnel: w893 -> [_ w903]
                tunnel: w892 -> [w894 w902]
                tunnel: [w894 w898] -> w891
                tunnel: w890 -> [_ w901]
                tunnel: w888 -> [_ w900]
                tunnel: w887 -> [_ w899]
                tunnel: w886 -> [_ w897]
                tunnel: w885 -> [_ w896]
                tunnel: w884 -> [_ w895]
                frame False {
                }
                frame True {
                  # "Ne se déplacer que si le moteur est actif"
                  n548 = case shown="False" w901 {
                    tunnel: w903 -> [w908 w940]
                    tunnel: w902 -> [w907 w939]
                    tunnel: [w909 w938] -> w898
                    tunnel: w900 -> [_ w937]
                    tunnel: w899 -> [w906 _]
                    tunnel: w897 -> [w905 _]
                    tunnel: w896 -> [_ w936]
                    tunnel: w895 -> [w904 w935]
                    frame False {
                      # "Déplacement en position miroir:\nbutée - ou ref"
                      n549 = case shown="True" w905 {
                        tunnel: [w915 w926] -> w909
                        tunnel: w908 -> [w914 w928]
                        tunnel: w907 -> [w912 w924]
                        tunnel: w906 -> [_ w927]
                        tunnel: w904 -> [w910 _]
                        frame False {
                          w916 = T7 1 items=["Mouvement Simple"=1, "Aller vers Cote"=2, "Va vers position de référence"=3] ("Type de mouvement")
                          # "Aller en butée si FAUX"
                          n550 = case shown="False" w910 {
                            tunnel: [u16 128 ("Ordre UC") u16 64 ("Ordre UC")] -> w911
                            frame False {
                              # "MIROIR\nPas d'inversion\nOrdre UC butée -"
                            }
                            frame True {
                              # "Ordre UC butée +"
                            }
                          }
                          n551 = local read "Adresse du PilMOT"() -> (w913:string)
                          n552 = Add(x=w914, y=1) -> (x+y=w920:i32)
                          n553 = call "FetchAxisSharedVars.vi"("error in (no error)"=w912, "Numéro d'Axe"=w920, "PilMOT Address"=w913) -> ("error out"=w918:errorcluster, "Sortie Variables d'Axes"=w917:T8)  [unwired: 7 in]
                          n554 = call "MovePilMot.vi"("Ordre UC"=w911, "Variables d'Axes"=w917, "error in (no error)"=w918, "Type de mouvement"=w916) -> ("error out"=w915:errorcluster)  [unwired: 11 in]
                        }
                        frame True {
                          w925 = u16 0 items=["Mouvement Relatif"=1, "Mouvement Absolu"=0] ("Mouvement Absolu/Relatif")
                          w930 = T7 2 items=["Mouvement Simple"=1, "Aller vers Cote"=2, "Va vers position de référence"=3] ("Type de mouvement")
                          # "Aller à la position de référence si VRAI"
                          n555 = local read "Adresse du PilMOT"() -> (w929:string)
                          n556 = Add(x=w928, y=1) -> (x+y=w934:i32)
                          n557 = call "FetchAxisSharedVars.vi"("error in (no error)"=w924, "Numéro d'Axe"=w934, "PilMOT Address"=w929) -> ("error out"=w932:errorcluster, "Sortie Variables d'Axes"=w931:T8)  [unwired: 7 in]
                          n558 = call "MovePilMot.vi"("Variables d'Axes"=w931, "Cote à atteindre"=w927, "Vitesse"=1500, "error in (no error)"=w932, "Type de mouvement"=w930, "Mouvement Absolu/Relatif"=w925) -> ("error out"=w926:errorcluster)  [unwired: 9 in]
                        }
                      }
                    }
                    frame True {
                      # "Déplacement en position atténuation:\nbutée + ou position de référence"
                      n559 = case shown="False" w936 {
                        tunnel: w940 -> [w952 w957]
                        tunnel: w939 -> [w951 w956]
                        tunnel: [w950 w958] -> w938
                        tunnel: w937 -> [_ w960]
                        tunnel: w935 -> [w942 _]
                        frame False {
                          w944 = T7 1 items=["Mouvement Simple"=1, "Aller vers Cote"=2, "Va vers position de référence"=3] ("Type de mouvement")
                          # "Aller en butée si FAUX"
                          n560 = case shown="True" w942 {
                            tunnel: [u16 64 ("Ordre UC") u16 128 ("Ordre UC")] -> w943
                            frame False {
                              # "ATTENUATEUR, \npas d'inversion\nOrdre UC butée +"
                            }
                            frame True {
                              # "Ordre UC butée -"
                            }
                          }
                          n561 = local read "Adresse du PilMOT"() -> (w947:string)
                          n562 = Add(x=w952, y=1) -> (x+y=w949:i32)
                          n563 = call "FetchAxisSharedVars.vi"("error in (no error)"=w951, "Numéro d'Axe"=w949, "PilMOT Address"=w947) -> ("error out"=w946:errorcluster, "Sortie Variables d'Axes"=w945:T8)  [unwired: 7 in]
                          n564 = call "MovePilMot.vi"("Ordre UC"=w943, "Variables d'Axes"=w945, "Vitesse"=1500, "error in (no error)"=w946, "Type de mouvement"=w944) -> ("error out"=w950:errorcluster)  [unwired: 10 in]
                        }
                        frame True {
                          w959 = u16 0 items=["Mouvement Relatif"=1, "Mouvement Absolu"=0] ("Mouvement Absolu/Relatif")
                          w961 = T7 2 items=["Mouvement Simple"=1, "Aller vers Cote"=2, "Va vers position de référence"=3] ("Type de mouvement")
                          # "Aller à la position de référence atténuation si VRAI"
                          n565 = local read "Adresse du PilMOT"() -> (w955:string)
                          n566 = Add(x=w957, y=1) -> (x+y=w965:i32)
                          n567 = call "FetchAxisSharedVars.vi"("error in (no error)"=w956, "Numéro d'Axe"=w965, "PilMOT Address"=w955) -> ("error out"=w963:errorcluster, "Sortie Variables d'Axes"=w962:T8)  [unwired: 7 in]
                          n568 = call "MovePilMot.vi"("Variables d'Axes"=w962, "Cote à atteindre"=w960, "error in (no error)"=w963, "Type de mouvement"=w961, "Mouvement Absolu/Relatif"=w959) -> ("error out"=w958:errorcluster)  [unwired: 10 in]
                        }
                      }
                    }
                  }
                }
              }
            }
            n569 = local write "error out"(w881) -> ()
          }
          event "HeNe Switch": Value Change {
            n570 = event-data() -> ()  [unwired: 1 in, 6 out]
            n571 = property on="HeNe in?" class="Bool (strict)"() -> ("Value"=w966:bool)  [unwired: 2 in, 2 out]
            n572 = case shown="True" w966 {
              tunnel: "Position Laser" -> [w973 _]
              tunnel: "Position HeNe" -> [_ w996]
              tunnel: "Inversion des butées HeNe" -> [w972 w995]
              tunnel: [w971 w994] -> w967
              frame False {
                # "Laser, butée ou\nposition de référence"
                n573 = case shown="False" w973 {
                  tunnel: w972 -> [w982 _]
                  tunnel: [w974 w985] -> w971
                  frame False {
                    w978 = T7 1 items=["Mouvement Simple"=1, "Aller vers Cote"=2, "Va vers position de référence"=3] ("Type de mouvement")
                    # "Si FAUX alors : En butée"
                    n574 = case shown="True" w982 {
                      tunnel: [u16 128 ("Ordre UC") u16 64 ("Ordre UC")] -> w975
                      frame False {
                        # "HeNe, \nsans inversion\nOrdre UC butée -"
                      }
                      frame True {
                        # "Laser, \ninversion\nOrdre UC butée +"
                      }
                    }
                    n575 = local read "Adresse du PilMOT"() -> (w981:string)
                    n576 = call "FetchAxisSharedVars.vi"("Numéro d'Axe"=u32 4, "PilMOT Address"=w981) -> ("error out"=w980:errorcluster, "Sortie Variables d'Axes"=w979:T8)  [unwired: 8 in]
                    n577 = call "MovePilMot.vi"("Ordre UC"=w975, "Variables d'Axes"=w979, "Vitesse"=1500, "error in (no error)"=w980, "Type de mouvement"=w978) -> ("error out"=w974:errorcluster)  [unwired: 10 in]
                  }
                  frame True {
                    w989 = u16 0 items=["Mouvement Relatif"=1, "Mouvement Absolu"=0] ("Mouvement Absolu/Relatif")
                    w991 = T7 2 items=["Mouvement Simple"=1, "Aller vers Cote"=2, "Va vers position de référence"=3] ("Type de mouvement")
                    # "si VRAI : Position de référence"
                    n578 = property on="Position de Référence Laser" class="DigNum (strict)"() -> ("Value"=w986:i32)  [unwired: 2 in, 2 out]
                    n579 = local read "Adresse du PilMOT"() -> (w990:string)
                    n580 = call "FetchAxisSharedVars.vi"("Numéro d'Axe"=u32 4, "PilMOT Address"=w990) -> ("error out"=w993:errorcluster, "Sortie Variables d'Axes"=w992:T8)  [unwired: 8 in]
                    n581 = call "MovePilMot.vi"("Variables d'Axes"=w992, "Cote à atteindre"=w986, "Vitesse"=1500, "error in (no error)"=w993, "Type de mouvement"=w991, "Mouvement Absolu/Relatif"=w989) -> ("error out"=w985:errorcluster)  [unwired: 9 in]
                  }
                }
              }
              frame True {
                # "HeNe, butée ou\nposition de référence"
                n582 = case shown="True" w996 {
                  tunnel: w995 -> [w997 _]
                  tunnel: [w998 w1008] -> w994
                  frame False {
                    w1002 = T7 1 items=["Mouvement Simple"=1, "Aller vers Cote"=2, "Va vers position de référence"=3] ("Type de mouvement")
                    # "Si FAUX alors : En butée"
                    n583 = case shown="True" w997 {
                      tunnel: [u16 64 ("Ordre UC") u16 128 ("Ordre UC")] -> w999
                      frame False {
                        # "HeNe, \npas d'inversion\nOrdre UC butée +"
                      }
                      frame True {
                        # "HeNe, \ninversion\nOrdre UC butée -"
                      }
                    }
                    n584 = local read "Adresse du PilMOT"() -> (w1005:string)
                    n585 = call "FetchAxisSharedVars.vi"("Numéro d'Axe"=u32 4, "PilMOT Address"=w1005) -> ("error out"=w1004:errorcluster, "Sortie Variables d'Axes"=w1003:T8)  [unwired: 8 in]
                    n586 = call "MovePilMot.vi"("Ordre UC"=w999, "Variables d'Axes"=w1003, "Vitesse"=1500, "error in (no error)"=w1004, "Type de mouvement"=w1002) -> ("error out"=w998:errorcluster)  [unwired: 10 in]
                  }
                  frame True {
                    w1012 = u16 0 items=["Mouvement Relatif"=1, "Mouvement Absolu"=0] ("Mouvement Absolu/Relatif")
                    w1014 = T7 2 items=["Mouvement Simple"=1, "Aller vers Cote"=2, "Va vers position de référence"=3] ("Type de mouvement")
                    # "Si VRAI alors : Position de référence"
                    n587 = property on="Position de Référence HeNe" class="DigNum (strict)"() -> ("Value"=w1009:i32)  [unwired: 2 in, 2 out]
                    n588 = local read "Adresse du PilMOT"() -> (w1013:string)
                    n589 = call "FetchAxisSharedVars.vi"("Numéro d'Axe"=u32 4, "PilMOT Address"=w1013) -> ("error out"=w1016:errorcluster, "Sortie Variables d'Axes"=w1015:T8)  [unwired: 8 in]
                    n590 = call "MovePilMot.vi"("Variables d'Axes"=w1015, "Cote à atteindre"=w1009, "Vitesse"=1500, "error in (no error)"=w1016, "Type de mouvement"=w1014, "Mouvement Absolu/Relatif"=w1012) -> ("error out"=w1008:errorcluster)  [unwired: 9 in]
                  }
                }
              }
            }
            n591 = property on="error out" class="Clust (strict)"("Value"=w967) -> ()  [unwired: 2 in, 2 out]
          }
          event "MT Déplacer +", "MT Deplacer -", "MT Butée +", "MT Butée -", "MT Origine ici": Value Change {
            n592 = event-data() -> ("NewVal"=w1017:bool)  [unwired: 1 in, 5 out]
            n593 = case shown="True" w1017 {
              frame False {
              }
              frame True {
                n594 = stacked-sequence {
                  frame #0 {
                    w1043 = T7 1 items=["Mouvement Simple"=1, "Aller vers Cote"=2, "Va vers position de référence"=3] ("Type de mouvement")
                    n595 = Boolean To (0,1)(Boolean="MT Déplacer +") -> (0, 1=w1041:i16)
                    n596 = Boolean To (0,1)(Boolean="MT Butée +") -> (0, 1=w1036:i16)
                    n597 = Boolean To (0,1)(Boolean="MT Deplacer -") -> (0, 1=w1038:i16)
                    n598 = Boolean To (0,1)(Boolean="MT Origine ici") -> (0, 1=w1032:i16)
                    n599 = Select(t=i16 16 ("y"), s="MT Origine ici", f=i16 0 ("y")) -> (s? t:f=w1021:i16)
                    n600 = Boolean To (0,1)(Boolean="MT Butée -") -> (0, 1=w1033:i16)
                    n601 = Multiply(x=w1041, y=i16 16) -> (x*y=w1030:i16)
                    n602 = Multiply(x=w1036, y=i16 64) -> (x*y=w1028:i16)
                    n603 = Multiply(x=w1038, y=i16 32) -> (x*y=w1029:i16)
                    n604 = Multiply(x=i16 2 ("y"), y=w1032) -> (x*y=w1026:i16)
                    n605 = Multiply(x=i16 128 ("y"), y=w1033) -> (x*y=w1027:i16)
                    n606 = Compound Arithmetic op=ADD(w1030, w1029, w1028, w1027, w1026) -> (w1025:i16)
                    n607 = local read "Adresse du PilMOT"() -> (w1046:string)
                    n608 = call "FetchAxisSharedVars.vi"("Numéro d'Axe"=u32 5, "PilMOT Address"=w1046) -> ("Sortie Variables d'Axes"=w1044:T8)  [unwired: 8 in, 1 out]
                    n609 = call "MovePilMot.vi"("Ordre UC"=w1025, "Variables d'Axes"=w1044, "Type de mouvement"=w1043, "Ordre Bloc"=w1021) -> ("error out"=w1020:errorcluster)  [unwired: 11 in]
                    n610 = local write "error out"(w1020) -> ()
                  }
                  frame #1 {
                    w1047 = FALSE
                    n611 = property on="MT Origine ici" class="Bool (strict)"("Value"=w1047) -> ()  [unwired: 2 in, 2 out]
                    n612 = property on="MT Butée +" class="Bool (strict)"("Value"=w1047) -> ()  [unwired: 2 in, 2 out]
                    n613 = property on="MT Deplacer -" class="Bool (strict)"("Value"=w1047) -> ()  [unwired: 2 in, 2 out]
                    n614 = property on="MT Déplacer +" class="Bool (strict)"("Value"=w1047) -> ()  [unwired: 2 in, 2 out]
                    n615 = property on="MT Butée -" class="Bool (strict)"("Value"=w1047) -> ()  [unwired: 2 in, 2 out]
                  }
                }
              }
            }
          }
          event "LR Origine ici", "LR Butée -", "LR Butée +", "LR Deplacer -", "LR Déplacer +": Value Change {
            n616 = event-data() -> ("NewVal"=w1048:bool)  [unwired: 1 in, 5 out]
            n617 = case shown="True" w1048 {
              frame False {
              }
              frame True {
                w1051 = T7 1 items=["Mouvement Simple"=1, "Aller vers Cote"=2, "Va vers position de référence"=3] ("Type de mouvement")
                n618 = Boolean To (0,1)(Boolean="LR Déplacer +") -> (0, 1=w1075:i16)
                n619 = Boolean To (0,1)(Boolean="LR Butée +") -> (0, 1=w1071:i16)
                n620 = Boolean To (0,1)(Boolean="LR Deplacer -") -> (0, 1=w1072:i16)
                n621 = Boolean To (0,1)(Boolean="LR Origine ici") -> (0, 1=w1067:i16)
                n622 = Select(t=i16 16 ("y"), s="LR Origine ici", f=i16 0 ("y")) -> (s? t:f=w1050:i16)
                n623 = Boolean To (0,1)(Boolean="LR Butée -") -> (0, 1=w1068:i16)
                n624 = Multiply(x=w1075, y=i16 16) -> (x*y=w1065:i16)
                n625 = Multiply(x=w1071, y=i16 64) -> (x*y=w1063:i16)
                n626 = Multiply(x=w1072, y=i16 32) -> (x*y=w1064:i16)
                n627 = Multiply(x=i16 2 ("y"), y=w1067) -> (x*y=w1061:i16)
                n628 = Multiply(x=i16 128 ("y"), y=w1068) -> (x*y=w1062:i16)
                n629 = Compound Arithmetic op=ADD(w1065, w1064, w1063, w1062, w1061) -> (w1052:i16)
                n630 = local read "Adresse du PilMOT"() -> (w1054:string)
                n631 = call "FetchAxisSharedVars.vi"("Numéro d'Axe"=u32 6, "PilMOT Address"=w1054) -> ("Sortie Variables d'Axes"=w1053:T8)  [unwired: 8 in, 1 out]
                n632 = call "MovePilMot.vi"("Ordre UC"=w1052, "Variables d'Axes"=w1053, "Type de mouvement"=w1051, "Ordre Bloc"=w1050) -> ("error out"=w1049:errorcluster)  [unwired: 11 in]
                n633 = local write "error out"(w1049) -> ()
              }
            }
          }
          event "Positions?": Value Change {
            n634 = event-data() -> ()  [unwired: 1 in, 6 out]
            n635 = local read "Axe3_Messages"() -> (w1080:u16)
            n636 = local read "Axe4_Messages"() -> (w1079:u16)
            n637 = local read "Axe2_Messages"() -> (w1081:u16)
            n638 = local read "Axe1_Messages"() -> (w1082:u16)
            n639 = Build Array(w1082, w1081, w1080, w1079) -> (w1078:u16[])
            n640 = for {
              tunnel: w1078 -> [w1092] mode=indexing
              i -> [w1089]
              n641 = call "U16To16Bits.vi"("Nombre à convertir"=w1092) -> ("Array of bits"=w1095:u16[])  [unwired: 10 in]
              n642 = Index Array(array=w1095, index #1=0 ("index"), index #2=1 ("index")) -> (element #1=w1091:u16, element #2=w1090:u16)
              n643 = Not Equal To 0?(x=w1091) -> (x != 0?=w1084:bool)
              n644 = Not Equal To 0?(x=w1090) -> (x != 0?=w1083:bool)
              n645 = local read "Butée N"() -> (w1088:bool[])
              n646 = local read "Butée P"() -> (w1086:bool[])
              n647 = Replace Array Subset(array=w1088, new element=w1083, index=w1089) -> (w1087:bool[])
              n648 = Replace Array Subset(array=w1086, new element=w1084, index=w1089) -> (w1085:bool[])
              n649 = local write "Butée N"(w1087) -> ()
              n650 = local write "Butée P"(w1085) -> ()
            }
          }
          event "HeNe en Butée?": Value Change {
            n651 = event-data() -> ()  [unwired: 1 in, 6 out]
            n652 = local read "Axe4_Messages"() -> (w1098:u16)
            n653 = call "U16To16Bits.vi"("Nombre à convertir"=w1098) -> ("Array of bits"=w1103:u16[])  [unwired: 10 in]
            n654 = Index Array(array=w1103, index #1=0 ("index"), index #2=1 ("index")) -> (element #1=w1100:u16, element #2=w1099:u16)
            n655 = Not Equal To 0?(x=w1100) -> (x != 0?=w1097:bool)
            n656 = Not Equal To 0?(x=w1099) -> (x != 0?=w1096:bool)
            n657 = local write "Butée N \n(HeNe)"(w1096) -> ()
            n658 = local write "Butée P \n(HeNe)"(w1097) -> ()
          }
          event "MT STOP mvt", "STOP Moteurs", "Ref. Tab STOP mvt", "STOP mvt", "LR STOP mvt": Value Change {
            n659 = event-data() -> ()  [unwired: 1 in, 6 out]
            n660 = call "Arret Urgence.vi"() -> ("error out"=w1105:errorcluster)  [unwired: 11 in]
            n661 = local write "error out"(w1105) -> ()
            n662 = Unbundle By Name(w1105) -> ("status"=w1104:bool)
          }
          event "stop": Value Change {
            n663 = event-data() -> ()  [unwired: 1 in, 6 out]
          }
        }
      }
    }
  }
